vi "Autonomous Independent.vi"() -> ()   [LabVIEW 2013]
doc: "This VI is called when autonomous begins, and will automatically be terminated when autonomous ends. You can carry out timed or sensor driven robot movement independently without needing to return to the caller."
uses:
  <vilib>/addons/Kinect/Skeleton Vertex Index.ctl
  Robot Global Data.vi
  <vilib>/addons/control/pid/pid.llb/PID (DBL).vi
  <vilib>/addons/control/pid/pid.llb/PID Control Input Filter (DBL).vi
  <vilib>/addons/control/pid/NI_PID_pid.lvlib
panel:
  out "Waveform Chart 4":dbl(graph)
  out "Waveform Chart 3":dbl(graph)
  out "Waveform Chart 2":dbl(graph)
  out "Waveform Chart":dbl(graph)
  out "Autonomous \nProgram":u32
  in  "Autonomous Mode":T1(tab)
  in  "When To Fire 1":dbl=5.0
  in  "auto 3 distance":dbl=110.0
  out "test auto":i32=13
  in  "stop delay":dbl=0.5
  out "Pause":bool
  out "State 2":i32
  in  "right turn angle 2":dbl=12.0
  in  "left turn angle 2":dbl=-12.0
  in  "auto 3 distance 3":dbl=92.0
  out "Turn Left":bool
  in  "Anti Rotate":T2={"proportional gain (Kc)"=0.03, "integral time (Ti, min)"=0.01, "derivative time (Td, min)"=0.003} {"derivative time (Td, min)" format="%.3f"; "integral time (Ti, min)" format="%.3f"; "proportional gain (Kc)" format="%.3f"}
  out "Autonomous state":u32
  in  "When To Start Firing":dbl=4.95
  in  "Abort Turn":dbl=1.5
  in  "When To Start Firing 2":dbl=4.95
  in  "right turn angle 3":dbl=10.0
  in  "left turn angle 3":dbl=-20.0
  in  "auto 3 distance 5":dbl=120.0
  out "State 3":i32
  out "Turn Left 2":bool
  in  "BackupLimit":dbl=12.0
  in  "BackupSpeed":dbl=0.3 format="%#_13g"
  in  "Catapult Down":dbl=1.5 format="%#_13g"
  in  "Fire Delay":dbl format="%#_13g"
  in  "Left Rotate":dbl=-0.75
  in  "Left Strafe":dbl=-0.25 format="%#_13g"
  in  "Fire Delay 2":dbl format="%#_13g"
  in  "Catapult Down 2":dbl=1.5 format="%#_13g"
  out "State 4":i32
  in  "auto 3 distance 6":dbl=148.0
  in  "Left Strafe 2":dbl=-0.25 format="%#_13g"
  in  "Left Rotate 2":dbl=-0.75
  in  "Abort Turn 2":dbl=1.5
  out "Turn Left 3":bool
  in  "right turn angle 4":dbl=10.0
  in  "left turn angle 4":dbl=-20.0
  in  "When To Start Firing 3":dbl=4.95
  in  "BackupSpeed 2":dbl=0.3 format="%#_13g"
  in  "BackupLimit 2":dbl=36.0
  in  "Slowdown Distance":dbl=48.0
  in  "Ball Drop Distance":dbl
  in  "Catapult Down 3":dbl=1.5 format="%#_13g"
  out "State 5":i32
  in  "Ball Drop Distance 2":dbl
  in  "Slowdown Distance 2":dbl=48.0
  in  "Abort Turn 3":dbl=1.5
  out "Turn Left 4":bool
  in  "BackupSpeed 3":dbl=0.3 format="%#_13g"
  in  "BackupLimit 3":dbl=36.0
  out "State":i32
  in  "auto 3 distance 4":dbl=117.5
  in  "Track PID":T2={"proportional gain (Kc)"=0.09, "integral time (Ti, min)"=0.003, "derivative time (Td, min)"=0.001} {"derivative time (Td, min)" format="%.3f"; "integral time (Ti, min)" format="%.3f"; "proportional gain (Kc)" format="%.3f"}
  in  "Rate Thresh":dbl=500.0 step=0.001
  in  "Threshhold 2":sgl(knob)=0.75626117 scale=0.0..2.0
  out "x > y?":bool
  out "x-y 2":cluster{"x":sgl, "y":sgl, "z":sgl}
  out "Y":sgl
  # "Auto 4 Settings that work\nAuto Distance 130\nSpeed 0.75"
  # "Be sure to right-click and choose Data Operations>>Make Current Value default if you want to save the array values with the VI"
  # "PID values to use for anti rotation\nP=.03\nI=.01\nD=.003"
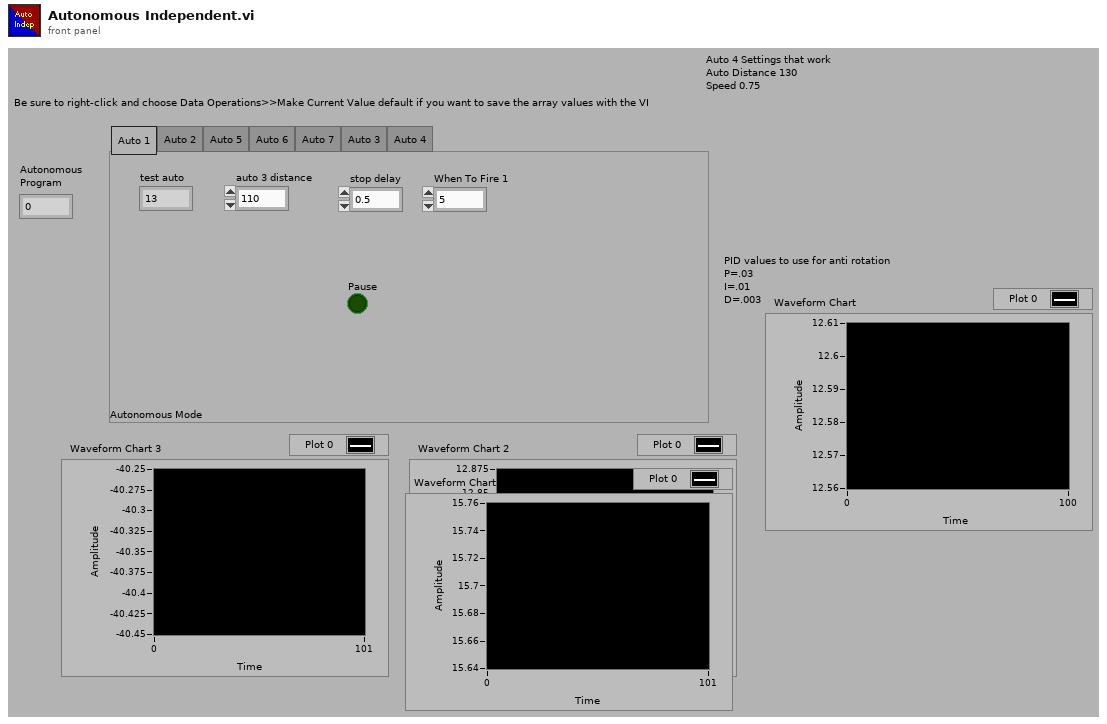
[diagram p1: front panel]
types:
  T1 = enum32{"Auto 1", "Auto 2", "Auto 5", "Auto 6", "Auto 7", "Auto 3", "Auto 4"}
  T2 = cluster{"proportional gain (Kc)":dbl, "integral time (Ti, min)":dbl, "derivative time (Td, min)":dbl}
  T3 = typedef "WPI_EncoderDevRef.ctl" = cluster{"DevStatus":errorcluster, "EncoderIndex":T4, "CounterIndex":T5, "DistancePerCount":dbl, "Decoding Type":T6}
  T4 = typedef "FPGA_EncoderIdx.ctl" = enum8{"Enc 0", "Enc 1", "Enc 2", "Enc 3", "Invalid"}
  T5 = typedef "FPGA_CounterCtrSystemIndex.ctl" = enum8{"Ctr 0", "Ctr 1", "Ctr 2", "Ctr 3", "Ctr 4", "Ctr 5", "Ctr 6", "Ctr 7", "Invalid"}
  T6 = typedef "WPI_EncoderType.ctl" = enum16{"1x", "2x", "4x"}
  T7 = typedef "WPI_GyroDevRef.ctl" = cluster{"DevStatus":errorcluster, "Analog Module":T8, "Analog Channel":T9, "Offset":dbl, "Gain (VoltsPerDegree/Second)":dbl}
  T8 = typedef "FPGA_TypedefAnalogModule.ctl" = enum16{"Analog Module 1", "Analog Module 2"}
  T9 = typedef "FPGA_AIChannel.ctl" = enum8{"AI 1", "AI 2", "AI 3", "AI 4", "AI 5", "AI 6", "AI 7", "AI 8", "Invalid"}
  T10 = typedef "WPI_AnalogChannelDevRef.ctl" = cluster{"DevStatus":errorcluster, "Analog Module":T8, "Analog Channel":T9}
  T11 = typedef "WPI_DigitalInputDevRef.ctl" = cluster{"DevStatus":errorcluster, "DIO Channel":T12, "Digital Module":T13}
  T12 = typedef "FPGA_DIOChannel.ctl" = enum8{"DIO 1", "DIO 2", "DIO 3", "DIO 4", "DIO 5", "DIO 6", "DIO 7", "DIO 8", "DIO 9", "DIO 10", "DIO 11", "DIO 12", "DIO 13", "DIO 14", "Invalid"}
  T13 = typedef "FPGA_TypedefDigitalModule.ctl" = enum16{"Digital Module 1", "Digital Module 2"}
  T14 = typedef "Skeleton Vertex Index.ctl" = i32
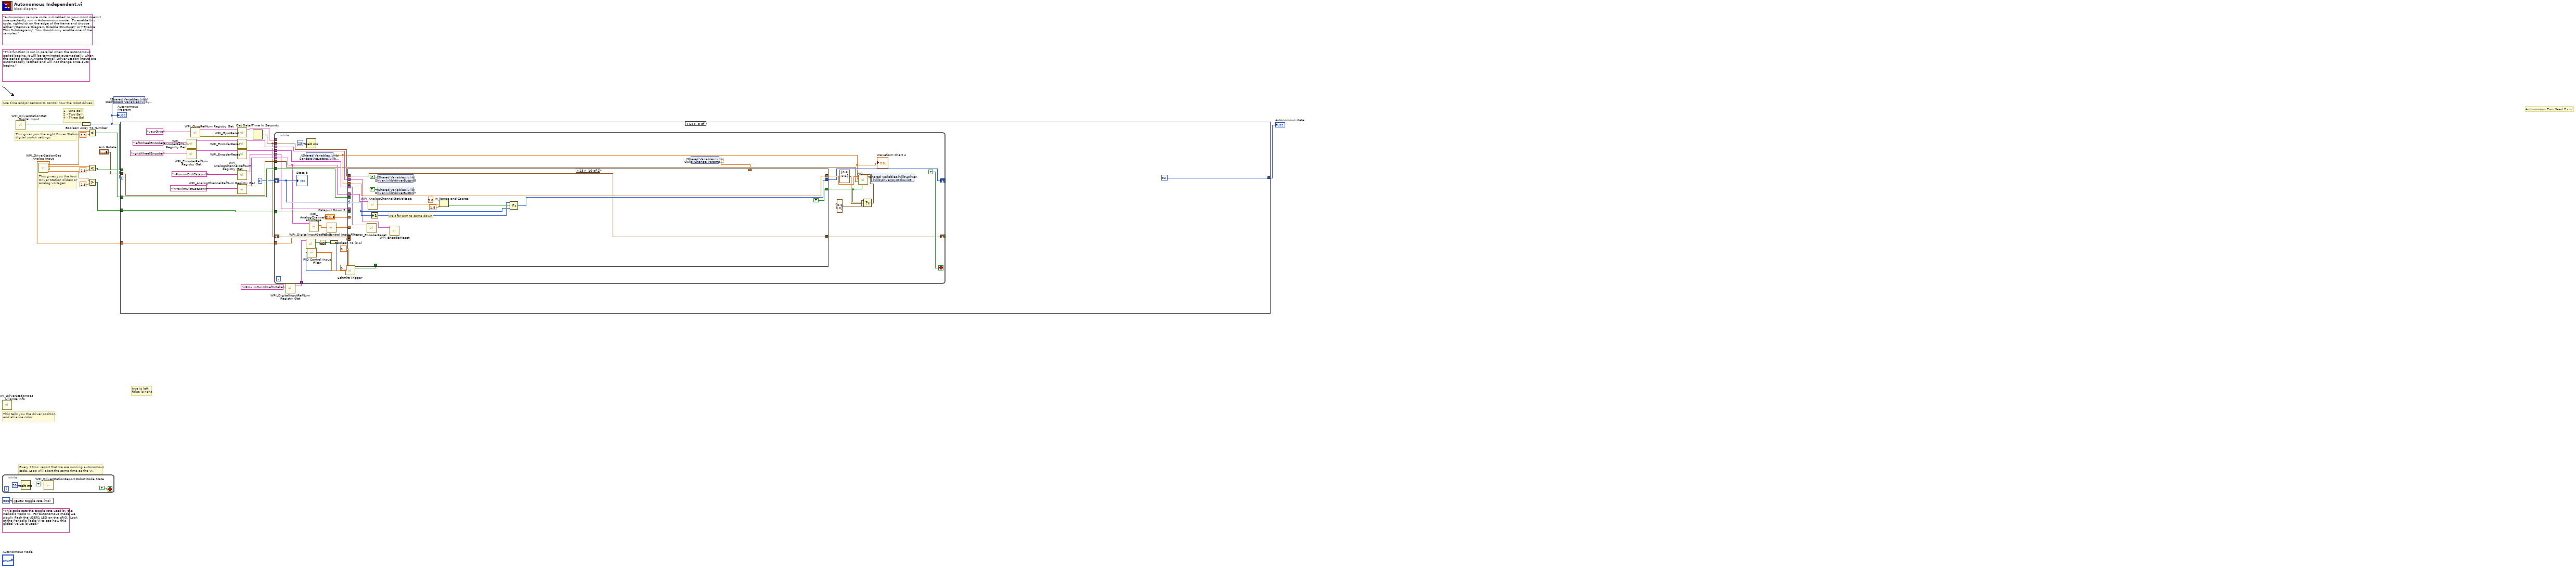
[diagram p0: block diagram]
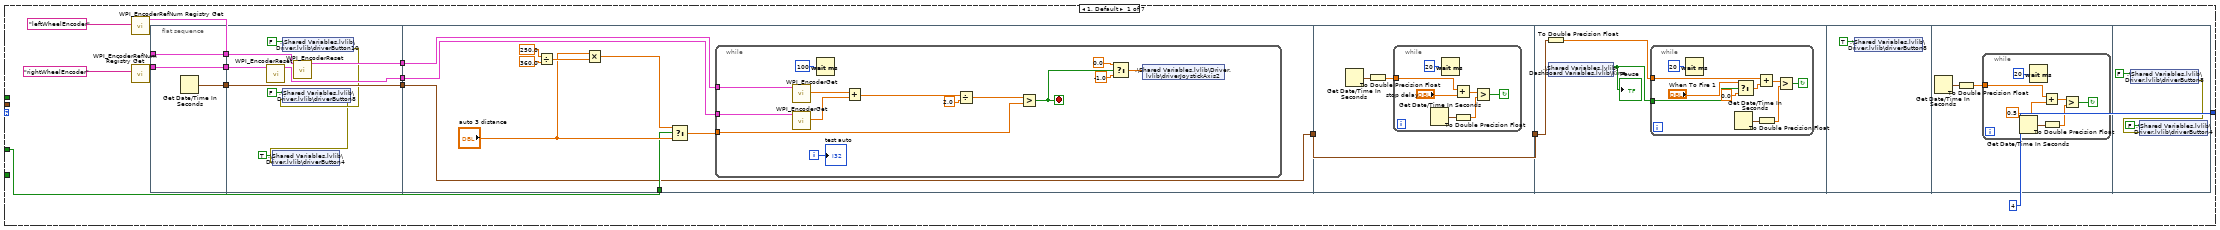
[diagram p2: hidden frame]
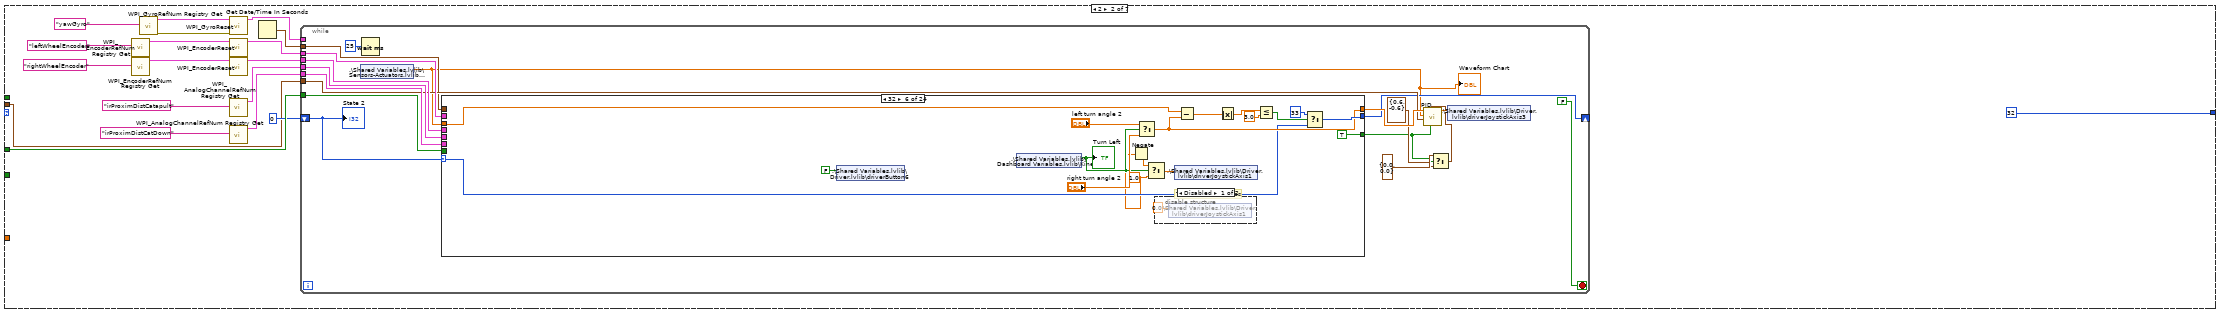
[diagram p3: hidden frame]
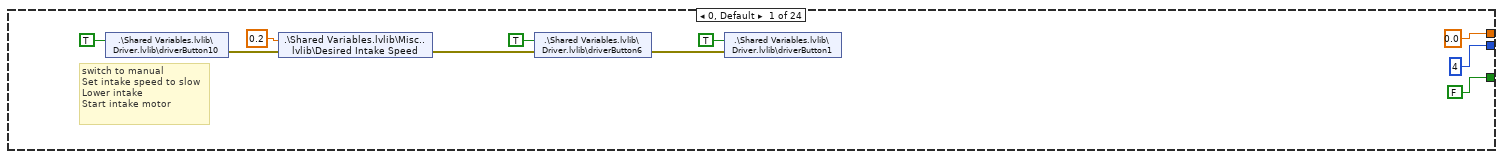
[diagram p4: hidden frame]
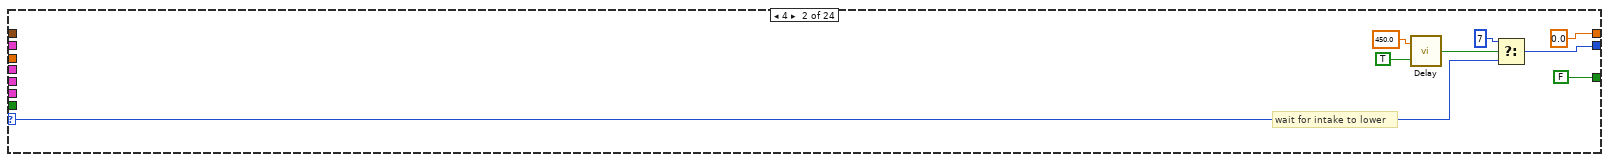
[diagram p5: hidden frame]
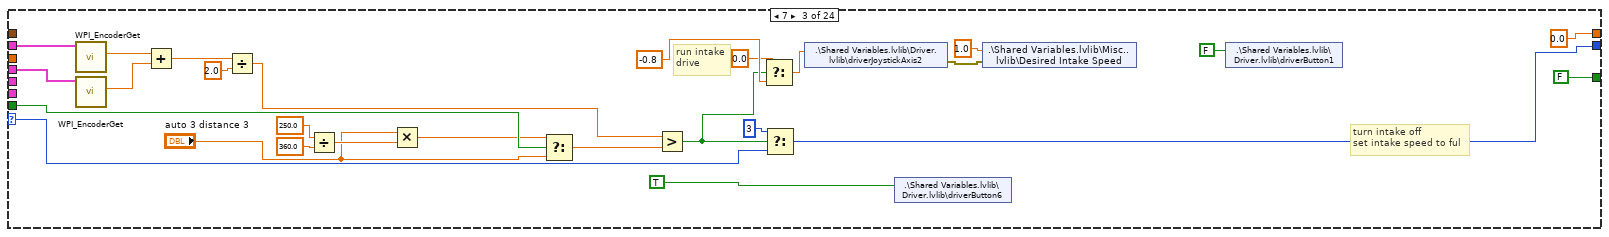
[diagram p6: hidden frame]
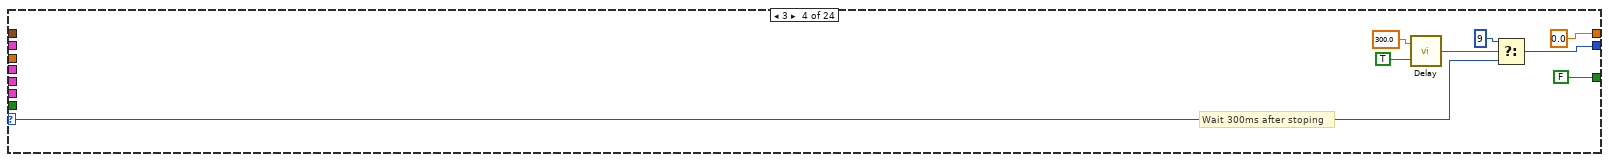
[diagram p7: hidden frame]
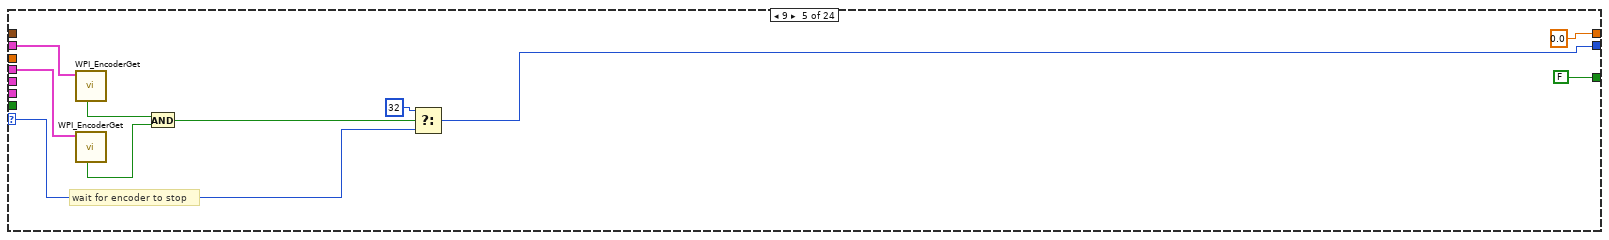
[diagram p8: hidden frame]
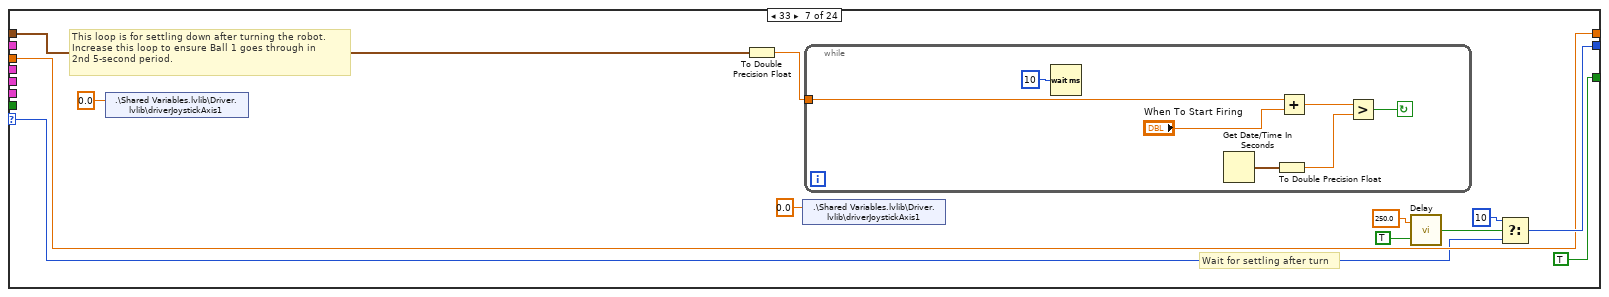
[diagram p10: hidden frame]
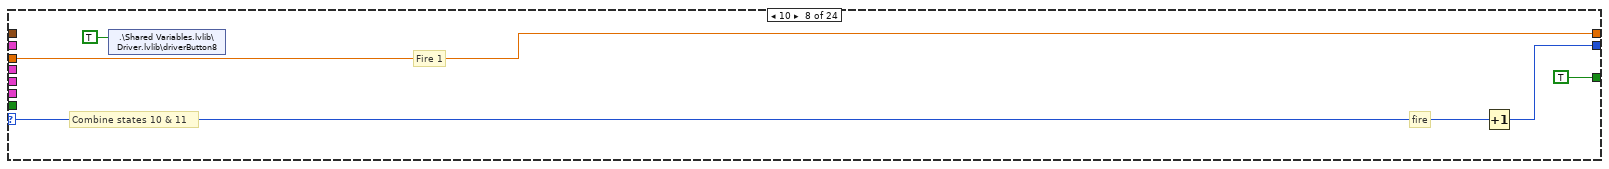
[diagram p11: hidden frame]
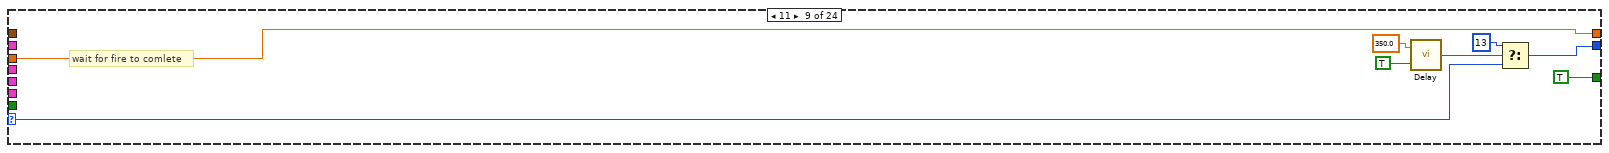
[diagram p12: hidden frame]
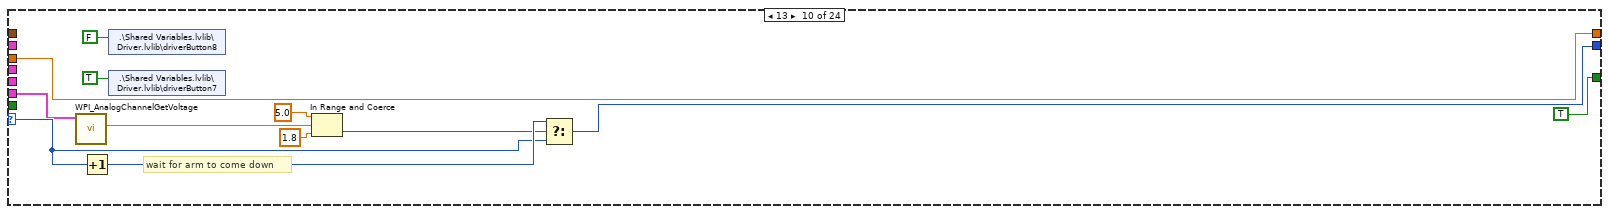
[diagram p13: hidden frame]
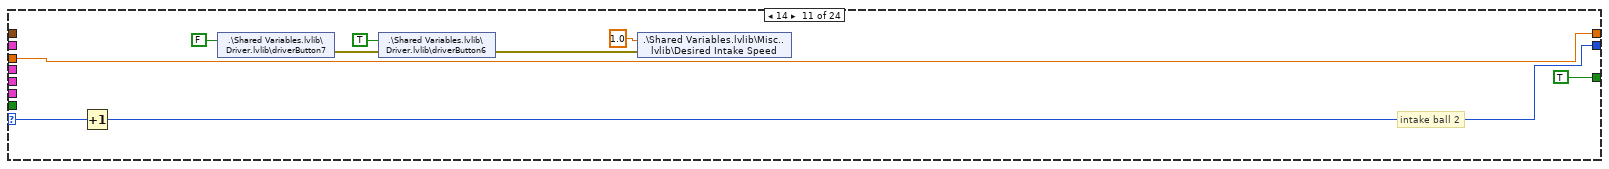
[diagram p14: hidden frame]
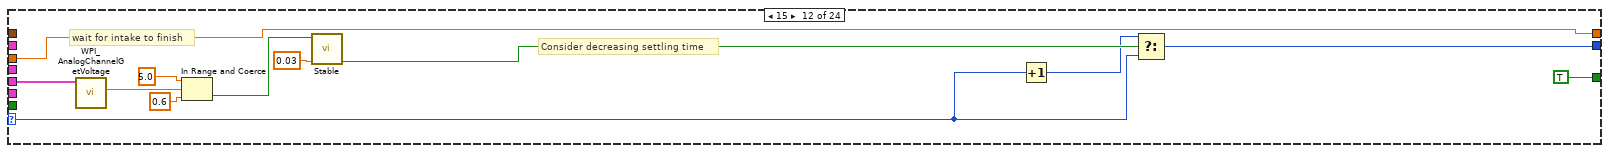
[diagram p15: hidden frame]
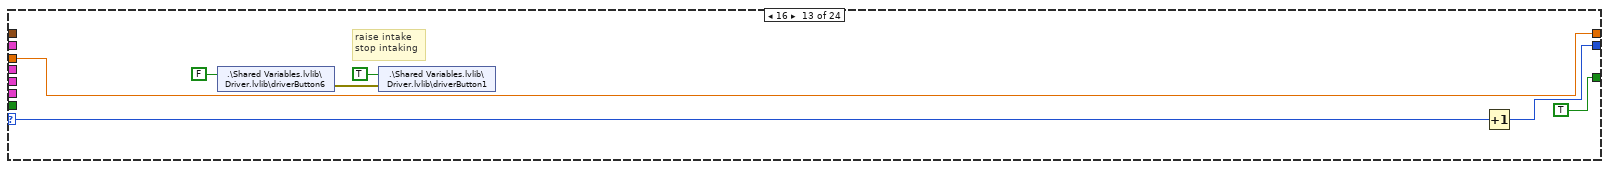
[diagram p16: hidden frame]
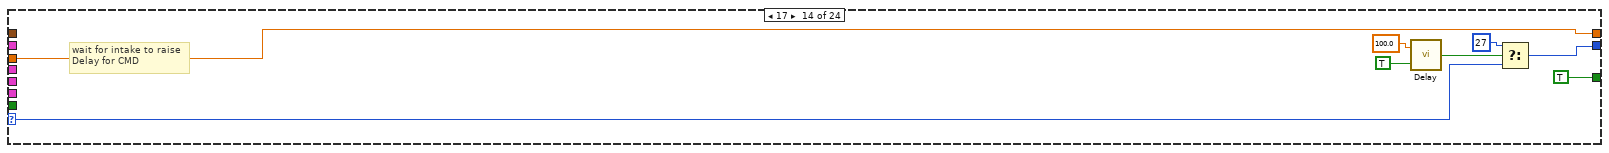
[diagram p17: hidden frame]
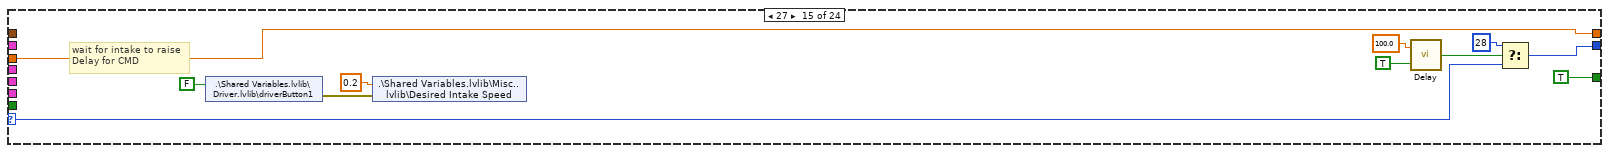
[diagram p18: hidden frame]
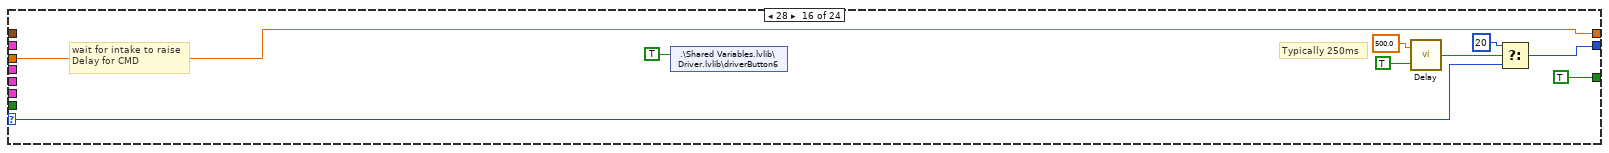
[diagram p19: hidden frame]
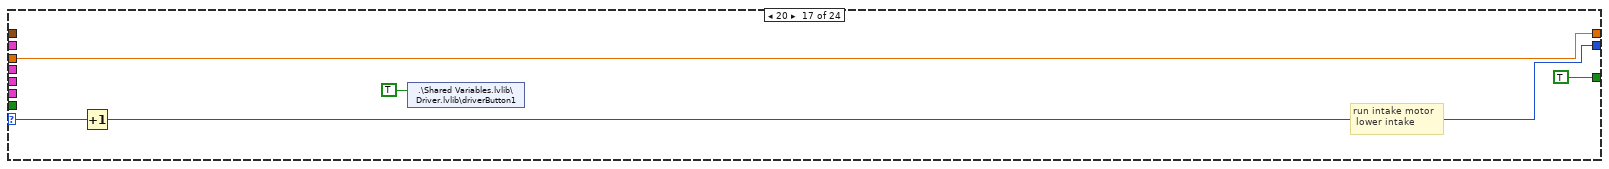
[diagram p20: hidden frame]
diagram:
  (unwired) "This code sets the toggle rate used by the Periodic Tasks VI.  For autonomous mode we slowly flash the USER1 LED on the cRIO.  Look at the Periodic Tasks VI to see how this global value is used."
  (unwired) "Autonomous sample code is disabled so your robot doesn't unexpectantly run in Autonomous mode.  To enable this code, right-click on the edge of the frame and choose either \"Remove Diagram Disable Structure\" or \"Enable This Subdiagram\". You should only enable one of the samples."
  (unwired) "This function is run in parallel when the autonomous period begins. It will be terminated automatically when the period ends.\n\nNote that all Driver Station inputs are automatically latched and will not change once auto begins."
  # "1 - One Ball\n2 - Two Ball\n4 - Three Bal"
  # "true is left\nfalse is right"
  # "Autonomous Two Need Fixin'"
  # "This gives you the eight Driver Station\ndigital switch settings"
  # "Every 20ms, report that we are running autonomous\ncode. Loop will abort the same time as the VI."
  # "Use time and/or sensors to control how the robot drives."
  # "This tells you the driver position\nand alliance color"
  # "This gives you the four\nDriver Station sliders or\nanalog voltages"
  n1 = call <vilib>:"WPI_DriverStationGet Alliance Info.vi"() -> ()  [unwired: 12 out]
  n2 = while {
    stop <- FALSE stop-if-true
    n3 = Wait (ms)(milliseconds to wait=u32 20) -> ()  [unwired: 1 out]
    n4 = call <vilib>:"WPI_DriverStationReport Robot Code State.vi"("Autonomous"=TRUE) -> ()  [unwired: 10 in, 1 out]
  }
  n5 = global write "Robot Global Data.vi" "LED toggle rate (ms)"(u32 500 ("LED ms toggle rate")) -> ()
  n6 = call <vilib>:"WPI_DriverStationGet Digital Input.vi"() -> ("Driver Station Digital Input (1-8)"=w14:bool[])  [unwired: 11 out]
  n7 = call <vilib>:"WPI_DriverStationGet Analog Input.vi"() -> ("Analog 4 (V)"=w3:dbl, "Analog 3 (V)"=w1:dbl, "Analog 2 (V)"=w7:dbl, "Analog 1 (V)"=w12:dbl)  [unwired: 8 out]
  n8 = Boolean Array To Number(Boolean array=w14) -> (number=w5:u32)
  "Autonomous \nProgram" <- w5
  n9 = Less?(x=w12, y=2.5) -> (x < y?=w10:bool)
  n10 = Less?(x=w7, y=2.5) -> (x < y?=w8:bool)
  n11 = Greater?(x=w3, y=2.5) -> (0:w2:bool)
  n12 = shared-variable ".\\Shared Variables.lvlib\\Dashboard Variables.lvlib\\Auto Mode"(w5) -> ()  [unwired: 1 in, 1 out]
  n13 = case shown="64" w5 {
    selector: w5 -> [_ _ _ _ _ _ w1912]
    tunnel: [4 32 32 32 32 16 w1912] -> w13
    tunnel: w10 -> [w25 w119 w398 w759 w1163 w1553 _]
    tunnel: w8 -> [_ _ _ _ _ w1564 _]
    tunnel: "Anti Rotate" -> [_ w107 w386 w747 w1151 w1559 _]
    tunnel: w2 -> [_ _ w382 w743 w1147 _ _]
    tunnel: w1 -> [_ _ w381 w742 w1146 _ _]
    frame 1, Default {
      n14 = call <vilib>:"WPI_EncoderRefNum Registry Get.vi"("refnum name"="leftWheelEncoder") -> ("EncoderDevRef"=w31:T3)  [unwired: 9 in, 1 out]
      n15 = call <vilib>:"WPI_EncoderRefNum Registry Get.vi"("refnum name"="rightWheelEncoder") -> ("EncoderDevRef"=w30:T3)  [unwired: 9 in, 1 out]
      n16 = flat-sequence {
        tunnel: w30 -> [w34]
        tunnel: w31 -> [w35]
        tunnel: [w35] -> w24
        tunnel: [w34] -> w23
        tunnel: [w33] -> w19
        tunnel: [w43] -> w27
        tunnel: [w42] -> w26
        tunnel: w24 -> [w45]
        tunnel: w23 -> [w44]
        tunnel: [w39] -> w20
        tunnel: w19 -> [w39]
        tunnel: w27 -> [w55]
        tunnel: w26 -> [w54]
        tunnel: w25 -> [w49]
        tunnel: [w46] -> w21
        tunnel: w20 -> [w46]
        tunnel: [w70] -> w22
        tunnel: w21 -> [w70]
        tunnel: w22 -> [w80]
        frame #0 {
          n17 = Get Date/Time In Seconds() -> (seconds since 1Jan1904=w33:timestamp)
        }
        frame #1 {
          n18 = call <vilib>:"WPI_EncoderReset.vi"("EncoderDevRef"=w44) -> ("EncoderDevRef"=w43:T3)  [unwired: 9 in, 1 out]
          n19 = shared-variable ".\\Shared Variables.lvlib\\Driver.lvlib\\driverButton10"(FALSE ("driverButton10")) -> (error out=w38:errorcluster)  [unwired: 1 in]
          n20 = shared-variable ".\\Shared Variables.lvlib\\Driver.lvlib\\driverButton8"(FALSE ("driverButton1"), error in=w38) -> (error out=w37:errorcluster)
          n21 = shared-variable ".\\Shared Variables.lvlib\\Driver.lvlib\\driverButton4"(TRUE ("driverButton4"), error in=w37) -> ()  [unwired: 1 out]
          n22 = call <vilib>:"WPI_EncoderReset.vi"("EncoderDevRef"=w45) -> ("EncoderDevRef"=w42:T3)  [unwired: 9 in, 1 out]
        }
        frame #2 {
          n23 = Divide(x=250.0, y=360.0) -> (x/y=w51:dbl)
          n24 = Multiply(x="auto 3 distance", y=w51) -> (x*y=w53:dbl)
          n25 = Select(t=w53, s=w49, f="auto 3 distance") -> (s? t:f=w48:dbl)
          n26 = while {
            tunnel: w55 -> [w63]
            tunnel: w54 -> [w62]
            tunnel: w48 -> [w56]
            i -> [w64]
            stop <- w66 stop-if-true
            n27 = call <vilib>:"WPI_EncoderGet.vi"("EncoderDevRef"=w62) -> ("Distance"=w61:dbl)  [unwired: 5 in, 5 out]
            n28 = call <vilib>:"WPI_EncoderGet.vi"("EncoderDevRef"=w63) -> ("Distance"=w60:dbl)  [unwired: 5 in, 5 out]
            n29 = Wait (ms)(milliseconds to wait=u32 100) -> ()  [unwired: 1 out]
            n30 = Add(x=w61, y=w60) -> (x+y=w59:dbl)
            n31 = Divide(x=w59, y=2.0) -> (x/y=w57:dbl)
            n32 = Greater?(x=w57, y=w56) -> (0:w66:bool)
            n33 = Select(t=0.0, s=w66, f=-1.0) -> (s? t:f=w67:dbl)
            n34 = shared-variable ".\\Shared Variables.lvlib\\Driver.lvlib\\driverJoystickAxis2"(w67) -> ()  [unwired: 1 in, 1 out]
            "test auto" <- w64
          }
        }
        frame #3 {
          n35 = Get Date/Time In Seconds() -> (seconds since 1Jan1904=w72:timestamp)
          n36 = To Double Precision Float(number=w72) -> (double precision float=w71:dbl)
          n37 = while {
            tunnel: w71 -> [w73]
            stop <- w76 continue-if-true
            n38 = Get Date/Time In Seconds() -> (seconds since 1Jan1904=w79:timestamp)
            n39 = Wait (ms)(milliseconds to wait=u32 20) -> ()  [unwired: 1 out]
            n40 = Add(x=w73, y="stop delay") -> (x+y=w78:dbl)
            n41 = To Double Precision Float(number=w79) -> (double precision float=w77:dbl)
            n42 = Greater?(x=w78, y=w77) -> (0:w76:bool)
          }
        }
        frame #4 {
          n43 = To Double Precision Float(number=w80) -> (double precision float=w82:dbl)
          n44 = shared-variable ".\\Shared Variables.lvlib\\Dashboard Variables.lvlib\\Kinect Status"() -> (w81:bool)  [unwired: 1 in, 1 out]
          "Pause" <- w81
          n45 = while {
            tunnel: w82 -> [w92]
            tunnel: w81 -> [w87]
            stop <- w88 continue-if-true
            n46 = Wait (ms)(milliseconds to wait=u32 20) -> ()  [unwired: 1 out]
            n47 = Get Date/Time In Seconds() -> (seconds since 1Jan1904=w91:timestamp)
            n48 = Select(t="When To Fire 1", s=w87, f=0.0) -> (s? t:f=w86:dbl)
            n49 = Add(x=w92, y=w86) -> (x+y=w90:dbl)
            n50 = To Double Precision Float(number=w91) -> (double precision float=w89:dbl)
            n51 = Greater?(x=w90, y=w89) -> (0:w88:bool)
          }
        }
        frame #5 {
          n52 = shared-variable ".\\Shared Variables.lvlib\\Driver.lvlib\\driverButton8"(TRUE ("driverButton1")) -> ()  [unwired: 1 in, 1 out]
        }
        frame #6 {
          n53 = Get Date/Time In Seconds() -> (seconds since 1Jan1904=w94:timestamp)
          n54 = To Double Precision Float(number=w94) -> (double precision float=w95:dbl)
          n55 = while {
            tunnel: w95 -> [w96]
            stop <- w99 continue-if-true
            n56 = Get Date/Time In Seconds() -> (seconds since 1Jan1904=w102:timestamp)
            n57 = Wait (ms)(milliseconds to wait=u32 20) -> ()  [unwired: 1 out]
            n58 = Add(x=w96, y=0.5 ("stop delay 2")) -> (x+y=w101:dbl)
            n59 = To Double Precision Float(number=w102) -> (double precision float=w100:dbl)
            n60 = Greater?(x=w101, y=w100) -> (0:w99:bool)
          }
        }
        frame #7 {
          n61 = shared-variable ".\\Shared Variables.lvlib\\Driver.lvlib\\driverButton8"(FALSE ("driverButton1")) -> (error out=w103:errorcluster)  [unwired: 1 in]
          n62 = shared-variable ".\\Shared Variables.lvlib\\Driver.lvlib\\driverButton4"(FALSE ("driverButton4"), error in=w103) -> ()  [unwired: 1 out]
        }
      }
    }
    frame 2 {
      n63 = call <vilib>:"WPI_EncoderRefNum Registry Get.vi"("refnum name"="leftWheelEncoder") -> ("EncoderDevRef"=w123:T3)  [unwired: 9 in, 1 out]
      n64 = call <vilib>:"WPI_EncoderRefNum Registry Get.vi"("refnum name"="rightWheelEncoder") -> ("EncoderDevRef"=w122:T3)  [unwired: 9 in, 1 out]
      n65 = call <vilib>:"WPI_GyroRefNum Registry Get.vi"("refnum name"="yawGyro") -> ("error out"=w110:errorcluster, "GyroDevRef"=w111:T7)  [unwired: 9 in]
      n66 = call <vilib>:"WPI_GyroReset.vi"("error in (no error)"=w110, "GyroDevRef"=w111) -> ("GyroDevRef"=w108:T7)  [unwired: 8 in, 1 out]
      n67 = call <vilib>:"WPI_EncoderReset.vi"("EncoderDevRef"=w123) -> ("EncoderDevRef"=w118:T3)  [unwired: 9 in, 1 out]
      n68 = call <vilib>:"WPI_EncoderReset.vi"("EncoderDevRef"=w122) -> ("EncoderDevRef"=w117:T3)  [unwired: 9 in, 1 out]
      n69 = call <vilib>:"WPI_AnalogChannelRefNum Registry Get.vi"("refnum name"="irProximDistCatapult") -> ("AIDeviceRef"=w116:T10)  [unwired: 9 in, 1 out]
      n70 = call <vilib>:"WPI_AnalogChannelRefNum Registry Get.vi"("refnum name"="irProximDistCatDown") -> ("AIDeviceRef"=w112:T10)  [unwired: 9 in, 1 out]
      n71 = Get Date/Time In Seconds() -> (seconds since 1Jan1904=w106:timestamp)
      n72 = while {
        tunnel: w119 -> [w142]
        tunnel: w118 -> [w141]
        tunnel: w117 -> [w140]
        tunnel: w116 -> [w137]
        shift-right: [w132] -> _
        shift-left: 0 -> [w136]
        tunnel: w112 -> [w135]
        tunnel: w108 -> [_]
        tunnel: w107 -> [w133]
        tunnel: w106 -> [w130]
        stop <- FALSE stop-if-true
        n73 = shared-variable ".\\Shared Variables.lvlib\\Sensors-Actuators.lvlib\\Gyro.lvlib\\yawGyro"() -> (w125:dbl)  [unwired: 1 in, 1 out]
        "Waveform Chart" <- w125
        n74 = Wait (ms)(milliseconds to wait=u32 25) -> ()  [unwired: 1 out]
        n75 = case shown="32" w136 {
          selector: w136 -> [_ w156 w172 w192 w205 w213 w231 w246 w252 w266 w275 w281 w294 w300 w311 w320 w328 w332 w342 w349 w358 w368 w371 w379]
          tunnel: [4 ("t") w158 w184 w191 w204 w220 w234 w245 w251 w265 w274 w279 w293 w299 w310 w319 w327 w331 w341 w348 w357 w369 w371 w379] -> w132
          tunnel: w142 -> [_ _ w187 _ _ _ _ _ _ _ _ _ _ _ _ _ _ _ _ _ _ _ _ _]
          tunnel: w141 -> [_ _ w186 _ w203 _ _ _ _ _ _ _ _ _ _ _ _ _ _ _ _ _ _ _]
          tunnel: w140 -> [_ _ w185 _ w202 _ _ _ _ _ _ _ _ _ _ _ _ _ _ _ _ _ _ _]
          tunnel: w137 -> [_ _ _ _ _ _ _ _ _ _ _ w288 _ _ _ _ _ _ _ _ _ _ _ _]
          tunnel: w135 -> [_ _ _ _ _ _ _ _ _ w264 _ _ _ _ _ _ _ _ _ _ _ w363 _ _]
          tunnel: [0.0 ("setpoint") 0.0 ("setpoint") 0.0 ("setpoint") 0.0 ("setpoint") 0.0 ("setpoint") w218 w233 w244 w250 w259 w271 w278 w290 w298 w309 w318 w326 w330 w338 w347 w355 w362 w373 w378] -> w134
          tunnel: w125 -> [_ _ _ _ _ w219 w233 w244 w250 w259 w271 w278 w290 w298 w309 w318 w326 w330 w338 w347 w355 w362 w373 w378]
          tunnel: [FALSE FALSE FALSE FALSE FALSE TRUE TRUE TRUE TRUE TRUE TRUE TRUE TRUE TRUE TRUE TRUE TRUE TRUE TRUE TRUE TRUE TRUE TRUE FALSE] -> w126
          tunnel: w130 -> [_ _ _ _ _ _ w225 _ _ _ _ _ _ _ _ _ _ _ _ _ _ _ _ _]
          frame 0, Default {
            # "switch to manual\nSet intake speed to slow\nLower intake\nStart intake motor"
            n76 = shared-variable ".\\Shared Variables.lvlib\\Driver.lvlib\\driverButton10"(TRUE ("driverButton10")) -> (error out=w144:errorcluster)  [unwired: 1 in]
            n77 = shared-variable ".\\Shared Variables.lvlib\\Misc..lvlib\\Desired Intake Speed"(0.2 ("Intake RPM"), error in=w144) -> (error out=w143:errorcluster)
            n78 = shared-variable ".\\Shared Variables.lvlib\\Driver.lvlib\\driverButton6"(TRUE ("driverButton6"), error in=w143) -> (error out=w146:errorcluster)
            n79 = shared-variable ".\\Shared Variables.lvlib\\Driver.lvlib\\driverButton1"(TRUE ("driverButton1"), error in=w146) -> ()  [unwired: 1 out]
          }
          frame 4 {
            # "wait for intake to lower"
            n80 = call "Delay.vi"("Timer Going?"=TRUE, "Time to Wait (ms)"=450.0) -> ("Time Up"=w159:bool)
            n81 = Select(t=7, s=w159, f=w156) -> (s? t:f=w158:i32)
          }
          frame 7 {
            # "turn intake off\nset intake speed to ful"
            # "run intake\ndrive"
            n82 = call <vilib>:"WPI_EncoderGet.vi"("EncoderDevRef"=w186) -> ("Distance"=w178:dbl)  [unwired: 5 in, 5 out]
            n83 = call <vilib>:"WPI_EncoderGet.vi"("EncoderDevRef"=w185) -> ("Distance"=w177:dbl)  [unwired: 5 in, 5 out]
            n84 = Add(x=w178, y=w177) -> (x+y=w176:dbl)
            n85 = Divide(x=w176, y=2.0) -> (x/y=w174:dbl)
            n86 = Divide(x=250.0, y=360.0) -> (x/y=w181:dbl)
            n87 = Multiply(x="auto 3 distance 3", y=w181) -> (x*y=w183:dbl)
            n88 = Select(t=w183, s=w187, f="auto 3 distance 3") -> (s? t:f=w173:dbl)
            n89 = Greater?(x=w174, y=w173) -> (0:w162:bool)
            n90 = Select(t=0.0, s=w162, f=-0.8 ("driverJoystickAxis2")) -> (s? t:f=w163:dbl)
            n91 = Select(t=3, s=w162, f=w172) -> (s? t:f=w184:i32)
            n92 = shared-variable ".\\Shared Variables.lvlib\\Driver.lvlib\\driverJoystickAxis2"(w163) -> (error out=w161:errorcluster)  [unwired: 1 in]
            n93 = shared-variable ".\\Shared Variables.lvlib\\Driver.lvlib\\driverButton6"(TRUE ("driverButton6")) -> ()  [unwired: 1 in, 1 out]
            n94 = shared-variable ".\\Shared Variables.lvlib\\Misc..lvlib\\Desired Intake Speed"(1.0 ("Desired Intake Speed"), error in=w161) -> ()  [unwired: 1 out]
            n95 = shared-variable ".\\Shared Variables.lvlib\\Driver.lvlib\\driverButton1"(FALSE ("driverButton1")) -> ()  [unwired: 1 in, 1 out]
          }
          frame 3 {
            # "Wait 300ms after stoping"
            n96 = call "Delay.vi"("Timer Going?"=TRUE, "Time to Wait (ms)"=300.0) -> ("Time Up"=w194:bool)
            n97 = Select(t=9 ("x"), s=w194, f=w192) -> (s? t:f=w191:i32)
          }
          frame 9 {
            # "wait for encoder to stop"
            n98 = call <vilib>:"WPI_EncoderGet.vi"("EncoderDevRef"=w203) -> ("Stopped"=w201:bool)  [unwired: 5 in, 5 out]
            n99 = call <vilib>:"WPI_EncoderGet.vi"("EncoderDevRef"=w202) -> ("Stopped"=w200:bool)  [unwired: 5 in, 5 out]
            n100 = And(x=w201, y=w200) -> (x .and. y?=w199:bool)
            n101 = Select(t=32, s=w199, f=w205) -> (s? t:f=w204:i32)
          }
          frame 32 {
            w207 = 1.0 ("f")
            # "Turn robot X degrees"
            n102 = shared-variable ".\\Shared Variables.lvlib\\Driver.lvlib\\driverButton6"(FALSE ("driverButton6")) -> ()  [unwired: 1 in, 1 out]
            n103 = shared-variable ".\\Shared Variables.lvlib\\Dashboard Variables.lvlib\\Kinect Status"() -> (w209:bool)  [unwired: 1 in, 1 out]
            "Turn Left" <- w209
            n104 = Negate(x=w207) -> (-x=w208:dbl)
            n105 = Select(t="left turn angle 2", s=w209, f="right turn angle 2") -> (s? t:f=w218:dbl)
            n106 = Select(t=w208, s=w209, f=w207) -> (s? t:f=w210:dbl)
            n107 = disable-structure shown="Disabled" {
              frame Disabled {
                n108 = shared-variable ".\\Shared Variables.lvlib\\Driver.lvlib\\driverJoystickAxis1"(0.0 ("driverJoystickAxis1")) -> ()  [unwired: 1 in, 1 out]
              }
              frame Enabled {
              }
            }
            n109 = shared-variable ".\\Shared Variables.lvlib\\Driver.lvlib\\driverJoystickAxis1"(w210) -> ()  [unwired: 1 in, 1 out]
            n110 = Subtract(x=w219, y=w218) -> (x-y=w217:dbl)
            n111 = Absolute Value(x=w217) -> (abs(x)=w216:dbl)
            n112 = Less Or Equal?(x=w216, y=3.0) -> (x <= y?=w214:bool)
            n113 = Select(t=33, s=w214, f=w213) -> (s? t:f=w220:i32)
          }
          frame 33 {
            # "This loop is for settling down after turning the robot.\nIncrease this loop to ensure Ball 1 goes through in \n2nd 5-second period."
            # "Wait for settling after turn"
            n114 = shared-variable ".\\Shared Variables.lvlib\\Driver.lvlib\\driverJoystickAxis1"(0.0 ("driverJoystickAxis1")) -> ()  [unwired: 1 in, 1 out]
            n115 = To Double Precision Float(number=w225) -> (double precision float=w226:dbl)
            n116 = shared-variable ".\\Shared Variables.lvlib\\Driver.lvlib\\driverJoystickAxis1"(0.0 ("driverJoystickAxis1")) -> ()  [unwired: 1 in, 1 out]
            n117 = while {
              tunnel: w226 -> [w236]
              stop <- w239 continue-if-true
              n118 = Wait (ms)(milliseconds to wait=u32 10) -> ()  [unwired: 1 out]
              n119 = Get Date/Time In Seconds() -> (seconds since 1Jan1904=w242:timestamp)
              n120 = To Double Precision Float(number=w242) -> (double precision float=w240:dbl)
              n121 = Add(x=w236, y="When To Start Firing") -> (x+y=w241:dbl)
              n122 = Greater?(x=w241, y=w240) -> (0:w239:bool)
            }
            n123 = call "Delay.vi"("Timer Going?"=TRUE, "Time to Wait (ms)"=250.0) -> ("Time Up"=w228:bool)
            n124 = Select(t=10, s=w228, f=w231) -> (s? t:f=w234:i32)
          }
          frame 10 {
            # "Combine states 10 & 11"
            # "Fire 1"
            # "fire"
            n125 = shared-variable ".\\Shared Variables.lvlib\\Driver.lvlib\\driverButton8"(TRUE ("driverButton8")) -> ()  [unwired: 1 in, 1 out]
            n126 = Increment(x=w246) -> (x+1=w245:i32)
          }
          frame 11 {
            # "wait for fire to comlete"
            n127 = call "Delay.vi"("Timer Going?"=TRUE, "Time to Wait (ms)"=350.0) -> ("Time Up"=w254:bool)
            n128 = Select(t=13, s=w254, f=w252) -> (s? t:f=w251:i32)
          }
          frame 13 {
            # "wait for arm to come down"
            n129 = call <vilib>:"WPI_AnalogChannelGetVoltage.vi"("AIDeviceRef"=w264) -> ("Voltage"=w263:dbl)  [unwired: 8 in, 2 out]
            n130 = Increment(x=w266) -> (x+1=w267:i32)
            n131 = shared-variable ".\\Shared Variables.lvlib\\Driver.lvlib\\driverButton8"(FALSE ("driverButton8")) -> ()  [unwired: 1 in, 1 out]
            n132 = shared-variable ".\\Shared Variables.lvlib\\Driver.lvlib\\driverButton7"(TRUE ("driverButton8")) -> ()  [unwired: 1 in, 1 out]
            n133 = In Range and Coerce(upper limit=5.0, x=w263, lower limit=1.8) -> (In Range?=w260:bool)  [unwired: 1 out]
            n134 = Select(t=w267, s=w260, f=w266) -> (s? t:f=w265:i32)
          }
          frame 14 {
            # "intake ball 2"
            n135 = Increment(x=w275) -> (x+1=w274:i32)
            n136 = shared-variable ".\\Shared Variables.lvlib\\Driver.lvlib\\driverButton7"(FALSE ("driverButton8")) -> (error out=w272:errorcluster)  [unwired: 1 in]
            n137 = shared-variable ".\\Shared Variables.lvlib\\Driver.lvlib\\driverButton6"(TRUE ("driverButton1"), error in=w272) -> (error out=w268:errorcluster)
            n138 = shared-variable ".\\Shared Variables.lvlib\\Misc..lvlib\\Desired Intake Speed"(1.0 ("Desired Intake Speed"), error in=w268) -> ()  [unwired: 1 out]
          }
          frame 15 {
            # "Consider decreasing settling time"
            # "wait for intake to finish"
            n139 = call <vilib>:"WPI_AnalogChannelGetVoltage.vi"("AIDeviceRef"=w288) -> ("Voltage"=w287:dbl)  [unwired: 8 in, 2 out]
            n140 = In Range and Coerce(upper limit=5.0, x=w287, lower limit=0.6) -> (In Range?=w284:bool)  [unwired: 1 out]
            n141 = call "Stable.vi"("Eval Period (sec)"=0.03, "Signal Input"=w284) -> ("Stable"=w282:bool)  [unwired: 9 in]
            n142 = Increment(x=w281) -> (x+1=w280:i32)
            n143 = Select(t=w280, s=w282, f=w281) -> (s? t:f=w279:i32)
          }
          frame 16 {
            # "raise intake\nstop intaking"
            n144 = shared-variable ".\\Shared Variables.lvlib\\Driver.lvlib\\driverButton6"(FALSE ("driverButton1")) -> (error out=w291:errorcluster)  [unwired: 1 in]
            n145 = shared-variable ".\\Shared Variables.lvlib\\Driver.lvlib\\driverButton1"(TRUE ("driverButton1"), error in=w291) -> ()  [unwired: 1 out]
            n146 = Increment(x=w294) -> (x+1=w293:i32)
          }
          frame 17 {
            # "wait for intake to raise\nDelay for CMD"
            n147 = call "Delay.vi"("Timer Going?"=TRUE, "Time to Wait (ms)"=100.0) -> ("Time Up"=w302:bool)
            n148 = Select(t=27, s=w302, f=w300) -> (s? t:f=w299:i32)
          }
          frame 27 {
            # "wait for intake to raise\nDelay for CMD"
            n149 = shared-variable ".\\Shared Variables.lvlib\\Driver.lvlib\\driverButton1"(FALSE ("driverButton1")) -> (error out=w304:errorcluster)  [unwired: 1 in]
            n150 = shared-variable ".\\Shared Variables.lvlib\\Misc..lvlib\\Desired Intake Speed"(0.2 ("Desired Intake Speed"), error in=w304) -> ()  [unwired: 1 out]
            n151 = call "Delay.vi"("Timer Going?"=TRUE, "Time to Wait (ms)"=100.0) -> ("Time Up"=w313:bool)
            n152 = Select(t=28, s=w313, f=w311) -> (s? t:f=w310:i32)
          }
          frame 28 {
            # "Typically 250ms"
            # "wait for intake to raise\nDelay for CMD"
            n153 = shared-variable ".\\Shared Variables.lvlib\\Driver.lvlib\\driverButton6"(TRUE ("driverButton1")) -> ()  [unwired: 1 in, 1 out]
            n154 = call "Delay.vi"("Timer Going?"=TRUE, "Time to Wait (ms)"=500.0) -> ("Time Up"=w322:bool)
            n155 = Select(t=20, s=w322, f=w320) -> (s? t:f=w319:i32)
          }
          frame 20 {
            # "run intake motor\n lower intake"
            n156 = Increment(x=w328) -> (x+1=w327:i32)
            n157 = shared-variable ".\\Shared Variables.lvlib\\Driver.lvlib\\driverButton1"(TRUE ("driverButton1")) -> ()  [unwired: 1 in, 1 out]
          }
          frame 21 {
            # "Consider decreasing settling time"
            # "wait for intake to lower\n(450ms)"
            n158 = Increment(x=w332) -> (x+1=w335:i32)
            n159 = call "Delay.vi"("Timer Going?"=TRUE, "Time to Wait (ms)"=450.0 ("Wait for Intake to Lower (450ms)")) -> ("Time Up"=w334:bool)
            n160 = Select(t=w335, s=w334, f=w332) -> (s? t:f=w331:i32)
          }
          frame 22 {
            # "stop running intake motor\nfire\nDe-Assert Lower Intake"
            n161 = Increment(x=w342) -> (x+1=w341:i32)
            n162 = shared-variable ".\\Shared Variables.lvlib\\Driver.lvlib\\driverButton1"(FALSE ("driverButton1")) -> (error out=w339:errorcluster)  [unwired: 1 in]
            n163 = shared-variable ".\\Shared Variables.lvlib\\Driver.lvlib\\driverButton6"(FALSE ("driverButton1"), error in=w339) -> (error out=w343:errorcluster)
            n164 = shared-variable ".\\Shared Variables.lvlib\\Driver.lvlib\\driverButton8"(TRUE ("driverButton1"), error in=w343) -> ()  [unwired: 1 out]
          }
          frame 23 {
            # "wait for fire"
            n165 = Increment(x=w349) -> (x+1=w352:i32)
            n166 = call "Delay.vi"("Timer Going?"=TRUE, "Time to Wait (ms)"=350.0) -> ("Time Up"=w351:bool)
            n167 = Select(t=w352, s=w351, f=w349) -> (s? t:f=w348:i32)
          }
          frame 24 {
            # "stop fire\nretract arm"
            n168 = shared-variable ".\\Shared Variables.lvlib\\Driver.lvlib\\driverButton8"(FALSE ("driverButton8")) -> (error out=w356:errorcluster)  [unwired: 1 in]
            n169 = shared-variable ".\\Shared Variables.lvlib\\Driver.lvlib\\driverButton7"(TRUE ("driverButton8"), error in=w356) -> ()  [unwired: 1 out]
            n170 = Increment(x=w358) -> (x+1=w357:i32)
          }
          frame 25 {
            # "wait for retract"
            n171 = call <vilib>:"WPI_AnalogChannelGetVoltage.vi"("AIDeviceRef"=w363) -> ("Voltage"=w367:dbl)  [unwired: 8 in, 2 out]
            n172 = In Range and Coerce(upper limit=5.0, x=w367, lower limit=1.5) -> (In Range?=w364:bool)  [unwired: 1 out]
            n173 = Increment(x=w368) -> (x+1=w370:i32)
            n174 = Select(t=w370, s=w364, f=w368) -> (s? t:f=w369:i32)
          }
          frame 26 {
            # "bring intake arm up\nEND AUTO"
            n175 = shared-variable ".\\Shared Variables.lvlib\\Driver.lvlib\\driverButton7"(FALSE ("driverButton8")) -> (error out=w374:errorcluster)  [unwired: 1 in]
            n176 = shared-variable ".\\Shared Variables.lvlib\\Driver.lvlib\\driverButton1"(TRUE ("driverButton1"), error in=w374) -> ()  [unwired: 1 out]
          }
          frame 29 {
            n177 = shared-variable ".\\Shared Variables.lvlib\\Driver.lvlib\\driverJoystickAxis1"(0.0 ("driverJoystickAxis1")) -> ()  [unwired: 1 in, 1 out]
          }
        }
        n178 = Select(t=cluster{"output high":dbl, "output low":dbl} {"output high"=0.0, "output low"=0.0} ("output range"), s=w126, f=cluster{"output high":dbl, "output low":dbl} {"output high"=0.6, "output low"=-0.6} ("output range")) -> (s? t:f=w127:cluster{"output high":dbl, "output low":dbl})
        n179 = call-poly <vilib>:"PID.vi"("reinitialize? (F)"=w126, "output range"=w127, "PID gains"=w133, "process variable"=w125, "setpoint"=w134) -> ("output"=w138:dbl)  [unwired: 5 in, 1 out]
        n180 = shared-variable ".\\Shared Variables.lvlib\\Driver.lvlib\\driverJoystickAxis3"(w138) -> ()  [unwired: 1 in, 1 out]
        "State 2" <- w136
      }
    }
    frame 16 {
      n181 = call <vilib>:"WPI_EncoderRefNum Registry Get.vi"("refnum name"="leftWheelEncoder") -> ("EncoderDevRef"=w402:T3)  [unwired: 9 in, 1 out]
      n182 = call <vilib>:"WPI_EncoderRefNum Registry Get.vi"("refnum name"="rightWheelEncoder") -> ("EncoderDevRef"=w401:T3)  [unwired: 9 in, 1 out]
      n183 = call <vilib>:"WPI_GyroRefNum Registry Get.vi"("refnum name"="yawGyro") -> ("error out"=w389:errorcluster, "GyroDevRef"=w390:T7)  [unwired: 9 in]
      n184 = call <vilib>:"WPI_GyroReset.vi"("error in (no error)"=w389, "GyroDevRef"=w390) -> ("GyroDevRef"=w387:T7)  [unwired: 8 in, 1 out]
      n185 = call <vilib>:"WPI_EncoderReset.vi"("EncoderDevRef"=w402) -> ("EncoderDevRef"=w397:T3)  [unwired: 9 in, 1 out]
      n186 = call <vilib>:"WPI_EncoderReset.vi"("EncoderDevRef"=w401) -> ("EncoderDevRef"=w396:T3)  [unwired: 9 in, 1 out]
      n187 = call <vilib>:"WPI_AnalogChannelRefNum Registry Get.vi"("refnum name"="irProximDistCatapult") -> ("AIDeviceRef"=w395:T10)  [unwired: 9 in, 1 out]
      n188 = call <vilib>:"WPI_AnalogChannelRefNum Registry Get.vi"("refnum name"="irProximDistCatDown") -> ("AIDeviceRef"=w391:T10)  [unwired: 9 in, 1 out]
      n189 = Get Date/Time In Seconds() -> (seconds since 1Jan1904=w383:timestamp)
      n190 = call <vilib>:"WPI_DigitalInputRefNum Registry Get.vi"("refnum name"="irProximSwitchLeftIntake") -> ("DigitalInputDevRef"=w384:T11)  [unwired: 9 in, 1 out]
      n191 = while {
        tunnel: w398 -> [w437]
        tunnel: w397 -> [w436]
        tunnel: w396 -> [w435]
        tunnel: w395 -> [w411]
        shift-right: [w429] -> _
        shift-left: 0 -> [w432]
        tunnel: w391 -> [w410]
        tunnel: w387 -> [_]
        tunnel: w386 -> [w430]
        tunnel: w383 -> [w427]
        tunnel: w384 -> [w419]
        shift-right: [w409] -> _
        shift-left: w383 -> [w408]
        tunnel: w382 -> [w405]
        tunnel: w381 -> [w404]
        stop <- FALSE stop-if-true
        n192 = shared-variable ".\\Shared Variables.lvlib\\Sensors-Actuators.lvlib\\Gyro.lvlib\\yawGyro"() -> (w422:dbl)  [unwired: 1 in, 1 out]
        "Waveform Chart 2" <- w422
        n193 = call <vilib>:"WPI_DigitalInputGetValue.vi"("DigitalInputDevRef"=w419) -> ("Value"=w420:bool)  [unwired: 8 in, 2 out]
        n194 = Wait (ms)(milliseconds to wait=u32 25) -> ()  [unwired: 1 out]
        n195 = call <vilib>:"WPI_AnalogChannelGetVoltage.vi"("AIDeviceRef"=w410) -> ("Voltage"=w412:dbl)  [unwired: 8 in, 2 out]
        n196 = Not(x=w420) -> (.not. x?=w418:bool)
        n197 = call-poly <vilib>:"PID Control Input Filter.vi"("input"=w412) -> ("output"=w421:dbl)  [unwired: 4 in]
        n198 = Boolean To (0,1)(Boolean=w418) -> (0, 1=w414:i16)
        n199 = call-poly <vilib>:"PID Control Input Filter.vi"("input"=w414) -> ("output"=w417:dbl)  [unwired: 4 in]
        n200 = call <userlib>:"Schmitt Trigger.vi"("lo"=sgl 0.1 ("High to Low\nTransition"), "in"=w417, "hi"=sgl 0.9 ("Low to High\nTransition")) -> ("out"=w413:bool)  [unwired: 1 out]
        n201 = case shown="13" w432 {
          selector: w432 -> [_ w455 w472 w493 w508 w531 w548 w563 w576 w592 w618 w633 w645 w652 w664 w674 w683 w688 w697 w712 w721 w732 w736]
          tunnel: [4 ("t") w457 w484 w492 w507 w537 w551 w562 w575 w591 w616 w631 w644 w651 w663 w673 w682 w687 w699 w711 w720 w733 w736] -> w429
          tunnel: w437 -> [_ _ w487 _ _ _ _ _ _ _ w596 _ _ _ _ _ _ _ _ _ _ _ _]
          tunnel: w436 -> [_ _ w486 _ w506 _ _ _ _ w580 w610 _ _ _ _ _ _ _ _ _ _ _ _]
          tunnel: w435 -> [_ _ w485 _ w505 _ _ _ _ w581 w609 _ _ _ _ _ _ _ _ _ _ _ _]
          tunnel: w410 -> [_ _ _ _ _ _ _ _ _ w590 _ _ _ _ _ _ _ _ _ _ _ w727 _]
          tunnel: [0.0 ("setpoint") 0.0 ("setpoint") 0.0 ("setpoint") 0.0 ("setpoint") 0.0 ("setpoint") w535 w550 w568 w574 w585 w622 w630 w641 w650 w662 w672 w681 w686 w701 w710 w718 w726 w738] -> w431
          tunnel: w422 -> [_ _ _ _ _ w536 w550 w568 w574 w585 w622 w630 w641 w650 w662 w672 w681 w686 w701 w710 w718 w726 w738]
          tunnel: [FALSE FALSE FALSE FALSE FALSE FALSE TRUE TRUE TRUE TRUE TRUE TRUE TRUE TRUE TRUE TRUE TRUE TRUE TRUE TRUE TRUE TRUE TRUE] -> w423
          tunnel: w427 -> [w440 w451 w460 w488 _ _ w542 w561 w571 w579 w603 w626 w639 w647 w656 w668 w678 w684 w694 w708 w716 w724 w735]
          tunnel: w421 -> [_ _ _ _ _ _ _ w564 _ _ _ _ _ _ _ _ _ _ w696 _ _ _ _]
          tunnel: w413 -> [_ _ _ _ _ _ _ _ _ _ w615 _ _ _ _ _ _ _ _ _ _ _ _]
          tunnel: w411 -> [_ _ _ _ _ _ _ _ _ _ _ w628 _ _ _ _ _ _ _ _ _ _ _]
          tunnel: [w440 w451 w460 w488 w498 w517 w542 w561 w571 w579 w603 w626 w639 w647 w656 w668 w678 w684 w694 w708 w716 w724 w735] -> w409
          tunnel: w408 -> [_ _ _ _ _ w517 _ _ _ _ _ _ _ _ _ _ _ _ _ _ _ _ _]
          tunnel: "Catapult Down" -> [_ _ _ _ _ _ _ w560 _ _ _ _ _ _ _ _ _ _ w693 _ _ _ _]
          tunnel: "Fire Delay" -> [_ _ _ _ _ _ _ _ w570 _ _ _ _ _ _ _ _ _ _ w707 _ _ _]
          tunnel: w405 -> [_ _ _ _ _ w515 _ _ _ _ _ _ _ _ _ _ _ _ _ _ _ _ _]
          tunnel: w404 -> [_ _ _ _ _ _ _ _ _ _ _ _ _ _ _ _ _ _ _ _ _ _ _]
          frame 0, Default {
            # "switch to manual\nSet intake speed to slow\nLower intake\nStart intake motor"
            n202 = shared-variable ".\\Shared Variables.lvlib\\Driver.lvlib\\driverButton10"(TRUE ("driverButton10")) -> (error out=w442:errorcluster)  [unwired: 1 in]
            n203 = shared-variable ".\\Shared Variables.lvlib\\Misc..lvlib\\Desired Intake Speed"(0.2 ("Intake RPM"), error in=w442) -> (error out=w441:errorcluster)
            n204 = shared-variable ".\\Shared Variables.lvlib\\Driver.lvlib\\driverButton6"(TRUE ("driverButton6"), error in=w441) -> (error out=w444:errorcluster)
            n205 = shared-variable ".\\Shared Variables.lvlib\\Driver.lvlib\\driverButton1"(TRUE ("driverButton1"), error in=w444) -> (error out=w438:errorcluster)
            n206 = shared-variable ".\\Shared Variables.lvlib\\Driver.lvlib\\driverButton7"(FALSE ("driverButton8"), error in=w438) -> ()  [unwired: 1 out]
          }
          frame 4 {
            # "wait for intake to lower"
            n207 = call "Delay.vi"("Timer Going?"=TRUE, "Time to Wait (ms)"=450.0) -> ("Time Up"=w458:bool)
            n208 = Select(t=7, s=w458, f=w455) -> (s? t:f=w457:i32)
          }
          frame 7 {
            # "turn intake off\nset intake speed to ful"
            # "run intake\ndrive"
            n209 = call <vilib>:"WPI_EncoderGet.vi"("EncoderDevRef"=w486) -> ("Distance"=w478:dbl)  [unwired: 5 in, 5 out]
            n210 = call <vilib>:"WPI_EncoderGet.vi"("EncoderDevRef"=w485) -> ("Distance"=w477:dbl)  [unwired: 5 in, 5 out]
            n211 = Add(x=w478, y=w477) -> (x+y=w476:dbl)
            n212 = Divide(x=w476, y=2.0) -> (x/y=w474:dbl)
            n213 = Divide(x=250.0, y=360.0) -> (x/y=w481:dbl)
            n214 = Multiply(x="auto 3 distance 5", y=w481) -> (x*y=w483:dbl)
            n215 = Select(t=w483, s=w487, f="auto 3 distance 5") -> (s? t:f=w473:dbl)
            n216 = Greater?(x=w474, y=w473) -> (0:w462:bool)
            n217 = Select(t=0.0, s=w462, f=-0.8 ("driverJoystickAxis2")) -> (s? t:f=w463:dbl)
            n218 = Select(t=3, s=w462, f=w472) -> (s? t:f=w484:i32)
            n219 = shared-variable ".\\Shared Variables.lvlib\\Driver.lvlib\\driverJoystickAxis2"(w463) -> (error out=w461:errorcluster)  [unwired: 1 in]
            n220 = shared-variable ".\\Shared Variables.lvlib\\Driver.lvlib\\driverButton6"(TRUE ("driverButton6")) -> ()  [unwired: 1 in, 1 out]
            n221 = shared-variable ".\\Shared Variables.lvlib\\Misc..lvlib\\Desired Intake Speed"(1.0 ("Desired Intake Speed"), error in=w461) -> ()  [unwired: 1 out]
            n222 = shared-variable ".\\Shared Variables.lvlib\\Driver.lvlib\\driverButton1"(FALSE ("driverButton1")) -> ()  [unwired: 1 in, 1 out]
          }
          frame 3 {
            # "Wait 300ms after stoping"
            n223 = call "Delay.vi"("Timer Going?"=TRUE, "Time to Wait (ms)"=300.0) -> ("Time Up"=w495:bool)
            n224 = Select(t=9 ("x"), s=w495, f=w493) -> (s? t:f=w492:i32)
          }
          frame 9 {
            # "wait for encoder to stop"
            n225 = call <vilib>:"WPI_EncoderGet.vi"("EncoderDevRef"=w506) -> ("Stopped"=w504:bool)  [unwired: 5 in, 5 out]
            n226 = call <vilib>:"WPI_EncoderGet.vi"("EncoderDevRef"=w505) -> ("Stopped"=w503:bool)  [unwired: 5 in, 5 out]
            n227 = And(x=w504, y=w503) -> (x .and. y?=w502:bool)
            n228 = Select(t=32, s=w502, f=w508) -> (s? t:f=w507:i32)
            n229 = shared-variable ".\\Shared Variables.lvlib\\Driver.lvlib\\driverButton6"(FALSE ("driverButton6")) -> ()  [unwired: 1 in, 1 out]
            n230 = Get Date/Time In Seconds() -> (seconds since 1Jan1904=w498:timestamp)
          }
          frame 32 {
            w527 = 1.0 ("f")
            # "Turn robot X degrees"
            n231 = To Double Precision Float(number=w517) -> (double precision float=w521:dbl)
            n232 = Get Date/Time In Seconds() -> (seconds since 1Jan1904=w523:timestamp)
            n233 = shared-variable ".\\Shared Variables.lvlib\\Driver.lvlib\\driverButton6"(FALSE ("driverButton6")) -> ()  [unwired: 1 in, 1 out]
            n234 = shared-variable ".\\Shared Variables.lvlib\\Driver.lvlib\\driverJoystickAxis2"(0.0 ("driverJoystickAxis2")) -> ()  [unwired: 1 in, 1 out]
            n235 = To Double Precision Float(number=w523) -> (double precision float=w522:dbl)
            n236 = Add(x=w521, y="Abort Turn") -> (x+y=w525:dbl)
            n237 = shared-variable ".\\Shared Variables.lvlib\\Dashboard Variables.lvlib\\Kinect Status"() -> (w516:bool)  [unwired: 1 in, 1 out]
            "Turn Left 2" <- w516
            n238 = Or(x=w516, y=w515) -> (x .or. y?=w514:bool)
            n239 = Less?(x=w525, y=w522) -> (x < y?=w520:bool)
            n240 = Select(t="Left Rotate", s=w514, f=0.0) -> (s? t:f=w512:dbl)
            n241 = Negate(x=w527) -> ()  [unwired: 1 out]
            n242 = Select(t="left turn angle 3", s=w514, f="right turn angle 3") -> (s? t:f=w535:dbl)
            n243 = Select(t="Left Strafe", s=w514, f=w527) -> (s? t:f=w528:dbl)
            n244 = disable-structure shown="Disabled" {
              frame Disabled {
                n245 = shared-variable ".\\Shared Variables.lvlib\\Driver.lvlib\\driverJoystickAxis1"(0.0 ("driverJoystickAxis1")) -> ()  [unwired: 1 in, 1 out]
              }
              frame Enabled {
              }
            }
            n246 = shared-variable ".\\Shared Variables.lvlib\\Driver.lvlib\\driverJoystickAxis1"(w528) -> ()  [unwired: 1 in, 1 out]
            n247 = Subtract(x=w536, y=w535) -> (x-y=w534:dbl)
            n248 = shared-variable ".\\Shared Variables.lvlib\\Driver.lvlib\\driverJoystickAxis3"(w512) -> ()  [unwired: 1 in, 1 out]
            n249 = Absolute Value(x=w534) -> (abs(x)=w533:dbl)
            n250 = Less Or Equal?(x=w533, y=3.0) -> (x <= y?=w519:bool)
            n251 = Or(x=w519, y=w520) -> (x .or. y?=w518:bool)
            n252 = Select(t=33, s=w518, f=w531) -> (s? t:f=w537:i32)
          }
          frame 33 {
            w541 = 0.0 ("driverJoystickAxis1")
            # "This loop is for settling down after turning the robot.\nIncrease this loop to ensure Ball 1 goes through in \n2nd 5-second period."
            # "Wait for settling after turn"
            n253 = shared-variable ".\\Shared Variables.lvlib\\Driver.lvlib\\driverJoystickAxis1"(0.0 ("driverJoystickAxis1")) -> ()  [unwired: 1 in, 1 out]
            n254 = To Double Precision Float(number=w542) -> (double precision float=w543:dbl)
            n255 = shared-variable ".\\Shared Variables.lvlib\\Driver.lvlib\\driverJoystickAxis3"(w541) -> ()  [unwired: 1 in, 1 out]
            n256 = shared-variable ".\\Shared Variables.lvlib\\Driver.lvlib\\driverJoystickAxis1"(w541) -> ()  [unwired: 1 in, 1 out]
            n257 = while {
              tunnel: w543 -> [w553]
              stop <- w556 continue-if-true
              n258 = Wait (ms)(milliseconds to wait=u32 10) -> ()  [unwired: 1 out]
              n259 = Get Date/Time In Seconds() -> (seconds since 1Jan1904=w559:timestamp)
              n260 = To Double Precision Float(number=w559) -> (double precision float=w557:dbl)
              n261 = Add(x=w553, y="When To Start Firing 2") -> (x+y=w558:dbl)
              n262 = Greater?(x=w558, y=w557) -> (0:w556:bool)
            }
            n263 = shared-variable ".\\Shared Variables.lvlib\\Driver.lvlib\\driverJoystickAxis2"(w541) -> ()  [unwired: 1 in, 1 out]
            n264 = call "Delay.vi"("Timer Going?"=TRUE, "Time to Wait (ms)"=250.0) -> ("Time Up"=w545:bool)
            n265 = Select(t=10, s=w545, f=w548) -> (s? t:f=w551:i32)
          }
          frame 10 {
            # "Combine states 10 & 11"
            # "Fire 1"
            # "fire"
            n266 = Increment(x=w563) -> (x+1=w566:i32)
            n267 = Greater Or Equal?(x=w560, y=w564) -> (x >= y?=w565:bool)
            n268 = shared-variable ".\\Shared Variables.lvlib\\Driver.lvlib\\driverButton8"(TRUE ("driverButton8")) -> ()  [unwired: 1 in, 1 out]
            n269 = Select(t=w566, s=w565, f=w563) -> (s? t:f=w562:i32)
          }
          frame 11 {
            # "wait for fire to comlete"
            n270 = call "Delay.vi"("Timer Going?"=TRUE, "Time to Wait (ms)"=w570) -> ("Time Up"=w577:bool)
            n271 = Select(t=13, s=w577, f=w576) -> (s? t:f=w575:i32)
          }
          frame 13 {
            # "wait for arm to come down"
            n272 = call <vilib>:"WPI_EncoderReset.vi"("EncoderDevRef"=w581) -> ()  [unwired: 9 in, 2 out]
            n273 = call <vilib>:"WPI_AnalogChannelGetVoltage.vi"("AIDeviceRef"=w590) -> ("Voltage"=w589:dbl)  [unwired: 8 in, 2 out]
            n274 = Increment(x=w592) -> (x+1=w593:i32)
            n275 = shared-variable ".\\Shared Variables.lvlib\\Driver.lvlib\\driverButton8"(FALSE ("driverButton8")) -> ()  [unwired: 1 in, 1 out]
            n276 = shared-variable ".\\Shared Variables.lvlib\\Driver.lvlib\\driverButton7"(TRUE ("driverButton8")) -> ()  [unwired: 1 in, 1 out]
            n277 = call <vilib>:"WPI_EncoderReset.vi"("EncoderDevRef"=w580) -> ()  [unwired: 9 in, 2 out]
            n278 = In Range and Coerce(upper limit=5.0, x=w589, lower limit=1.8) -> (In Range?=w586:bool)  [unwired: 1 out]
            n279 = Select(t=w593, s=w586, f=w592) -> (s? t:f=w591:i32)
          }
          frame 14 {
            # "intake ball 2"
            n280 = call <vilib>:"WPI_EncoderGet.vi"("EncoderDevRef"=w609) -> ("Distance"=w613:dbl)  [unwired: 5 in, 5 out]
            n281 = call <vilib>:"WPI_EncoderGet.vi"("EncoderDevRef"=w610) -> ("Distance"=w614:dbl)  [unwired: 5 in, 5 out]
            n282 = Increment(x=w618) -> (x+1=w617:i32)
            n283 = Add(x=w614, y=w613) -> (x+y=w612:dbl)
            n284 = shared-variable ".\\Shared Variables.lvlib\\Driver.lvlib\\driverButton7"(FALSE ("driverButton8")) -> (error out=w623:errorcluster)  [unwired: 1 in]
            n285 = Divide(x=w612, y=2.0) -> (x/y=w602:dbl)
            n286 = Absolute Value(x=w602) -> (abs(x)=w601:dbl)
            n287 = Divide(x=250.0, y=360.0) -> (x/y=w598:dbl)
            n288 = shared-variable ".\\Shared Variables.lvlib\\Driver.lvlib\\driverButton6"(TRUE ("driverButton1"), error in=w623) -> (error out=w619:errorcluster)
            n289 = Multiply(x="BackupLimit", y=w598) -> (x*y=w600:dbl)
            n290 = Select(t=w600, s=w596, f="BackupLimit") -> (s? t:f=w594:dbl)
            n291 = Greater Or Equal?(x=w601, y=w594) -> (x >= y?=w608:bool)
            n292 = Or(x=w608, y=w615) -> (x .or. y?=w607:bool)
            n293 = Select(t=w617, s=w607, f=w618) -> (s? t:f=w616:i32)
            n294 = Select(t=0.0, s=w607, f="BackupSpeed") -> (s? t:f=w604:dbl)
            n295 = shared-variable ".\\Shared Variables.lvlib\\Driver.lvlib\\driverJoystickAxis2"(w604) -> ()  [unwired: 1 in, 1 out]
            n296 = shared-variable ".\\Shared Variables.lvlib\\Misc..lvlib\\Desired Intake Speed"(1.0 ("Desired Intake Speed"), error in=w619) -> ()  [unwired: 1 out]
          }
          frame 15 {
            # "Consider decreasing settling time"
            # "wait for intake to finish"
            n297 = call <vilib>:"WPI_AnalogChannelGetVoltage.vi"("AIDeviceRef"=w628) -> ("Voltage"=w627:dbl)  [unwired: 8 in, 2 out]
            n298 = In Range and Coerce(upper limit=5.0, x=w627, lower limit=0.6) -> (In Range?=w636:bool)  [unwired: 1 out]
            n299 = call "Stable.vi"("Eval Period (sec)"=0.03, "Signal Input"=w636) -> ("Stable"=w634:bool)  [unwired: 9 in]
            n300 = Increment(x=w633) -> (x+1=w632:i32)
            n301 = Select(t=w632, s=w634, f=w633) -> (s? t:f=w631:i32)
          }
          frame 16 {
            # "raise intake\nstop intaking"
            n302 = shared-variable ".\\Shared Variables.lvlib\\Driver.lvlib\\driverButton6"(FALSE ("driverButton1")) -> (error out=w642:errorcluster)  [unwired: 1 in]
            n303 = shared-variable ".\\Shared Variables.lvlib\\Driver.lvlib\\driverButton1"(TRUE ("driverButton1"), error in=w642) -> ()  [unwired: 1 out]
            n304 = Increment(x=w645) -> (x+1=w644:i32)
          }
          frame 17 {
            # "wait for intake to raise\nDelay for CMD"
            n305 = call "Delay.vi"("Timer Going?"=TRUE, "Time to Wait (ms)"=100.0) -> ("Time Up"=w654:bool)
            n306 = Select(t=27, s=w654, f=w652) -> (s? t:f=w651:i32)
          }
          frame 27 {
            # "wait for intake to raise\nDelay for CMD"
            n307 = shared-variable ".\\Shared Variables.lvlib\\Driver.lvlib\\driverButton1"(FALSE ("driverButton1")) -> (error out=w657:errorcluster)  [unwired: 1 in]
            n308 = shared-variable ".\\Shared Variables.lvlib\\Misc..lvlib\\Desired Intake Speed"(0.2 ("Desired Intake Speed"), error in=w657) -> ()  [unwired: 1 out]
            n309 = call "Delay.vi"("Timer Going?"=TRUE, "Time to Wait (ms)"=100.0) -> ("Time Up"=w666:bool)
            n310 = Select(t=28, s=w666, f=w664) -> (s? t:f=w663:i32)
          }
          frame 28 {
            # "Typically 250ms"
            # "wait for intake to raise\nDelay for CMD"
            n311 = shared-variable ".\\Shared Variables.lvlib\\Driver.lvlib\\driverButton6"(TRUE ("driverButton1")) -> ()  [unwired: 1 in, 1 out]
            n312 = call "Delay.vi"("Timer Going?"=TRUE, "Time to Wait (ms)"=500.0) -> ("Time Up"=w676:bool)
            n313 = Select(t=20, s=w676, f=w674) -> (s? t:f=w673:i32)
          }
          frame 20 {
            # "run intake motor\n lower intake"
            n314 = Increment(x=w683) -> (x+1=w682:i32)
            n315 = shared-variable ".\\Shared Variables.lvlib\\Driver.lvlib\\driverButton1"(TRUE ("driverButton1")) -> ()  [unwired: 1 in, 1 out]
          }
          frame 21 {
            # "Consider decreasing settling time"
            # "wait for intake to lower\n(450ms)"
            n316 = Increment(x=w688) -> (x+1=w691:i32)
            n317 = call "Delay.vi"("Timer Going?"=TRUE, "Time to Wait (ms)"=450.0 ("Wait for Intake to Lower (450ms)")) -> ("Time Up"=w690:bool)
            n318 = Select(t=w691, s=w690, f=w688) -> (s? t:f=w687:i32)
          }
          frame 22 {
            # "stop running intake motor\nfire\nDe-Assert Lower Intake"
            n319 = Increment(x=w697) -> (x+1=w698:i32)
            n320 = Greater Or Equal?(x=w693, y=w696) -> (x >= y?=w695:bool)
            n321 = Select(t=w698, s=w695, f=w697) -> (s? t:f=w699:i32)
            n322 = shared-variable ".\\Shared Variables.lvlib\\Driver.lvlib\\driverButton1"(FALSE ("driverButton1")) -> (error out=w702:errorcluster)  [unwired: 1 in]
            n323 = shared-variable ".\\Shared Variables.lvlib\\Driver.lvlib\\driverButton6"(FALSE ("driverButton1"), error in=w702) -> (error out=w704:errorcluster)
            n324 = shared-variable ".\\Shared Variables.lvlib\\Driver.lvlib\\driverButton8"(TRUE ("driverButton1"), error in=w704) -> ()  [unwired: 1 out]
          }
          frame 23 {
            # "wait for fire"
            n325 = Increment(x=w712) -> (x+1=w715:i32)
            n326 = call "Delay.vi"("Timer Going?"=TRUE, "Time to Wait (ms)"=w707) -> ("Time Up"=w714:bool)
            n327 = Select(t=w715, s=w714, f=w712) -> (s? t:f=w711:i32)
          }
          frame 24 {
            # "stop fire\nretract arm"
            n328 = shared-variable ".\\Shared Variables.lvlib\\Driver.lvlib\\driverButton8"(FALSE ("driverButton8")) -> (error out=w719:errorcluster)  [unwired: 1 in]
            n329 = shared-variable ".\\Shared Variables.lvlib\\Driver.lvlib\\driverButton7"(TRUE ("driverButton8"), error in=w719) -> ()  [unwired: 1 out]
            n330 = Increment(x=w721) -> (x+1=w720:i32)
          }
          frame 25 {
            # "wait for retract"
            n331 = call <vilib>:"WPI_AnalogChannelGetVoltage.vi"("AIDeviceRef"=w727) -> ("Voltage"=w731:dbl)  [unwired: 8 in, 2 out]
            n332 = In Range and Coerce(upper limit=5.0, x=w731, lower limit=1.5) -> (In Range?=w728:bool)  [unwired: 1 out]
            n333 = Increment(x=w732) -> (x+1=w734:i32)
            n334 = Select(t=w734, s=w728, f=w732) -> (s? t:f=w733:i32)
          }
          frame 26 {
            # "bring intake arm up\nEND AUTO"
            n335 = shared-variable ".\\Shared Variables.lvlib\\Driver.lvlib\\driverButton7"(FALSE ("driverButton8")) -> (error out=w739:errorcluster)  [unwired: 1 in]
            n336 = shared-variable ".\\Shared Variables.lvlib\\Driver.lvlib\\driverButton1"(TRUE ("driverButton1"), error in=w739) -> ()  [unwired: 1 out]
          }
        }
        n337 = Select(t=cluster{"output high":dbl, "output low":dbl} {"output high"=0.0, "output low"=0.0} ("output range"), s=w423, f=cluster{"output high":dbl, "output low":dbl} {"output high"=0.6, "output low"=-0.6} ("output range")) -> (s? t:f=w424:cluster{"output high":dbl, "output low":dbl})
        n338 = call-poly <vilib>:"PID.vi"("reinitialize? (F)"=w423, "output range"=w424, "PID gains"=w430, "process variable"=w422, "setpoint"=w431) -> ("output"=w433:dbl)  [unwired: 5 in, 1 out]
        n339 = shared-variable ".\\Shared Variables.lvlib\\Driver.lvlib\\driverJoystickAxis3"(w433) -> ()  [unwired: 1 in, 1 out]
        "State 3" <- w432
      }
    }
    frame 32 {
      n340 = call <vilib>:"WPI_EncoderRefNum Registry Get.vi"("refnum name"="leftWheelEncoder") -> ("EncoderDevRef"=w763:T3)  [unwired: 9 in, 1 out]
      n341 = call <vilib>:"WPI_EncoderRefNum Registry Get.vi"("refnum name"="rightWheelEncoder") -> ("EncoderDevRef"=w762:T3)  [unwired: 9 in, 1 out]
      n342 = call <vilib>:"WPI_GyroRefNum Registry Get.vi"("refnum name"="yawGyro") -> ("error out"=w750:errorcluster, "GyroDevRef"=w751:T7)  [unwired: 9 in]
      n343 = call <vilib>:"WPI_GyroReset.vi"("error in (no error)"=w750, "GyroDevRef"=w751) -> ("GyroDevRef"=w748:T7)  [unwired: 8 in, 1 out]
      n344 = call <vilib>:"WPI_EncoderReset.vi"("EncoderDevRef"=w763) -> ("EncoderDevRef"=w758:T3)  [unwired: 9 in, 1 out]
      n345 = call <vilib>:"WPI_EncoderReset.vi"("EncoderDevRef"=w762) -> ("EncoderDevRef"=w757:T3)  [unwired: 9 in, 1 out]
      n346 = call <vilib>:"WPI_AnalogChannelRefNum Registry Get.vi"("refnum name"="irProximDistCatapult") -> ("AIDeviceRef"=w756:T10)  [unwired: 9 in, 1 out]
      n347 = call <vilib>:"WPI_AnalogChannelRefNum Registry Get.vi"("refnum name"="irProximDistCatDown") -> ("AIDeviceRef"=w752:T10)  [unwired: 9 in, 1 out]
      n348 = Get Date/Time In Seconds() -> (seconds since 1Jan1904=w744:timestamp)
      n349 = call <vilib>:"WPI_DigitalInputRefNum Registry Get.vi"("refnum name"="irProximSwitchLeftIntake") -> ("DigitalInputDevRef"=w745:T11)  [unwired: 9 in, 1 out]
      n350 = while {
        tunnel: w759 -> [w798]
        tunnel: w758 -> [w797]
        tunnel: w757 -> [w796]
        tunnel: w756 -> [w772]
        shift-right: [w790] -> _
        shift-left: 0 -> [w793]
        tunnel: w752 -> [w771]
        tunnel: w748 -> [_]
        tunnel: w747 -> [w791]
        tunnel: w744 -> [w788]
        tunnel: w745 -> [w780]
        shift-right: [w770] -> _
        shift-left: w744 -> [w769]
        tunnel: w743 -> [w766]
        tunnel: w742 -> [w765]
        stop <- FALSE stop-if-true
        n351 = shared-variable ".\\Shared Variables.lvlib\\Sensors-Actuators.lvlib\\Gyro.lvlib\\yawGyro"() -> (w783:dbl)  [unwired: 1 in, 1 out]
        "Waveform Chart 3" <- w783
        n352 = call <vilib>:"WPI_DigitalInputGetValue.vi"("DigitalInputDevRef"=w780) -> ("Value"=w781:bool)  [unwired: 8 in, 2 out]
        n353 = Wait (ms)(milliseconds to wait=u32 25) -> ()  [unwired: 1 out]
        n354 = call <vilib>:"WPI_AnalogChannelGetVoltage.vi"("AIDeviceRef"=w771) -> ("Voltage"=w773:dbl)  [unwired: 8 in, 2 out]
        n355 = Not(x=w781) -> (.not. x?=w779:bool)
        n356 = call-poly <vilib>:"PID Control Input Filter.vi"("input"=w773) -> ("output"=w782:dbl)  [unwired: 4 in]
        n357 = Boolean To (0,1)(Boolean=w779) -> (0, 1=w775:i16)
        n358 = call-poly <vilib>:"PID Control Input Filter.vi"("input"=w775) -> ("output"=w778:dbl)  [unwired: 4 in]
        n359 = call <userlib>:"Schmitt Trigger.vi"("lo"=sgl 0.1 ("High to Low\nTransition"), "in"=w778, "hi"=sgl 0.9 ("Low to High\nTransition")) -> ("out"=w774:bool)  [unwired: 1 out]
        n360 = case shown="10" w793 {
          selector: w793 -> [_ w816 w857 w879 w894 w923 w938 w953 w966 w982 w1008 w1023 w1035 w1042 w1054 w1064 w1073 w1078 w1087 w1102 w1111 w1122 w1126 w1144]
          tunnel: [4 ("t") w818 w866 w878 w893 w927 w941 w952 w965 w981 w1006 w1021 w1034 w1041 w1053 w1063 w1072 w1077 w1089 w1101 w1110 w1123 w1125 w1144] -> w790
          tunnel: w798 -> [_ _ w831 _ _ _ _ _ _ _ w986 _ _ _ _ _ _ _ _ _ _ _ _ _]
          tunnel: w797 -> [_ _ w868 _ w892 _ _ _ _ w970 w1000 _ _ _ _ _ _ _ _ _ _ _ _ _]
          tunnel: w796 -> [_ _ w867 _ w891 _ _ _ _ w971 w999 _ _ _ _ _ _ _ _ _ _ _ _ _]
          tunnel: w771 -> [_ _ _ _ _ _ _ _ _ w980 _ _ _ _ _ _ _ _ _ _ _ w1117 _ _]
          tunnel: [0.0 ("setpoint") 0.0 ("setpoint") 0.0 ("setpoint") 0.0 ("setpoint") 0.0 ("setpoint") w898 w940 w958 w964 w975 w1012 w1020 w1031 w1040 w1052 w1062 w1071 w1076 w1091 w1100 w1108 w1116 w1133 w1143] -> w792
          tunnel: w783 -> [_ _ _ _ _ w901 w940 w958 w964 w975 w1012 w1020 w1031 w1040 w1052 w1062 w1071 w1076 w1091 w1100 w1108 w1116 w1133 w1143]
          tunnel: [FALSE FALSE FALSE FALSE FALSE FALSE TRUE TRUE TRUE TRUE TRUE TRUE TRUE TRUE TRUE TRUE TRUE TRUE TRUE TRUE TRUE TRUE TRUE TRUE] -> w784
          tunnel: w788 -> [w801 w812 _ w874 _ _ w932 w951 w961 w969 w993 w1016 w1029 w1037 w1046 w1058 w1068 w1074 w1084 w1098 w1106 w1114 w1131 w1141]
          tunnel: w782 -> [_ _ _ _ _ _ _ w954 _ _ _ _ _ _ _ _ _ _ w1086 _ _ _ _ _]
          tunnel: w774 -> [_ _ _ _ _ _ _ _ _ _ w1005 _ _ _ _ _ _ _ _ _ _ _ _ _]
          tunnel: w772 -> [_ _ _ _ _ _ _ _ _ _ _ w1018 _ _ _ _ _ _ _ _ _ _ _ _]
          tunnel: [w801 w812 w821 w874 w884 w910 w932 w951 w961 w969 w993 w1016 w1029 w1037 w1046 w1058 w1068 w1074 w1084 w1098 w1106 w1114 w1131 w1141] -> w770
          tunnel: w769 -> [_ _ _ _ _ w910 _ _ _ _ _ _ _ _ _ _ _ _ _ _ _ _ _ _]
          tunnel: "Catapult Down 2" -> [_ _ _ _ _ _ _ w950 _ _ _ _ _ _ _ _ _ _ w1083 _ _ _ _ _]
          tunnel: "Fire Delay 2" -> [_ _ _ _ _ _ _ _ w960 _ _ _ _ _ _ _ _ _ _ w1097 _ _ _ _]
          tunnel: w766 -> [_ _ _ _ _ w908 _ _ _ _ _ _ _ _ _ _ _ _ _ _ _ _ _ _]
          tunnel: w765 -> [_ _ _ _ _ _ _ _ _ _ _ _ _ _ _ _ _ _ _ _ _ _ _ _]
          frame 0, Default {
            # "switch to manual\nSet intake speed to slow\nLower intake\nStart intake motor"
            n361 = shared-variable ".\\Shared Variables.lvlib\\Driver.lvlib\\driverButton10"(TRUE ("driverButton10")) -> (error out=w803:errorcluster)  [unwired: 1 in]
            n362 = shared-variable ".\\Shared Variables.lvlib\\Misc..lvlib\\Desired Intake Speed"(0.2 ("Intake RPM"), error in=w803) -> (error out=w802:errorcluster)
            n363 = shared-variable ".\\Shared Variables.lvlib\\Driver.lvlib\\driverButton6"(TRUE ("driverButton6"), error in=w802) -> (error out=w805:errorcluster)
            n364 = shared-variable ".\\Shared Variables.lvlib\\Driver.lvlib\\driverButton1"(TRUE ("driverButton1"), error in=w805) -> (error out=w799:errorcluster)
            n365 = shared-variable ".\\Shared Variables.lvlib\\Driver.lvlib\\driverButton7"(FALSE ("driverButton8"), error in=w799) -> ()  [unwired: 1 out]
          }
          frame 4 {
            # "wait for intake to lower"
            n366 = call "Delay.vi"("Timer Going?"=TRUE, "Time to Wait (ms)"=450.0) -> ("Time Up"=w819:bool)
            n367 = Select(t=7, s=w819, f=w816) -> (s? t:f=w818:i32)
          }
          frame 7 {
            # "turn intake off\nset intake speed to ful"
            n368 = call <vilib>:"WPI_EncoderGet.vi"("EncoderDevRef"=w868) -> ("Distance"=w861:dbl)  [unwired: 5 in, 5 out]
            n369 = call <vilib>:"WPI_EncoderGet.vi"("EncoderDevRef"=w867) -> ("Distance"=w860:dbl)  [unwired: 5 in, 5 out]
            n370 = Add(x=w861, y=w860) -> (x+y=w859:dbl)
            n371 = Divide(x=w859, y=2.0) -> (x/y=w824:dbl)
            n372 = Divide(x=250.0, y=360.0) -> (x/y=w828:dbl)
            n373 = Multiply(x="auto 3 distance 6", y=w828) -> (x*y=w865:dbl)
            n374 = Multiply(x=w828, y="Slowdown Distance") -> (x*y=w849:dbl)
            n375 = Select(t=w849, s=w831, f="Slowdown Distance") -> (s? t:f=w846:dbl)
            n376 = Multiply(x=w828, y="Ball Drop Distance") -> (x*y=w830:dbl)
            n377 = Select(t=w830, s=w831, f="Ball Drop Distance") -> (s? t:f=w827:dbl)
            n378 = Select(t=w865, s=w831, f="auto 3 distance 6") -> (s? t:f=w826:dbl)
            n379 = Subtract(x=w826, y=w846) -> (x-y=w847:dbl)
            n380 = Subtract(x=w826, y=w827) -> (x-y=w825:dbl)
            n381 = Greater?(x=w824, y=w847) -> (0:w833:bool)
            n382 = Greater?(x=w824, y=w825) -> (0:w823:bool)
            n383 = Greater?(x=w824, y=w826) -> (0:w851:bool)
            n384 = disable-structure shown="Disabled" {
              disable-tunnel: w851 -> [w870 _]
              disable-tunnel: [w869 _] -> w850
              frame Disabled {
                # "run intake\ndrive"
                n385 = Select(t=0.0, s=w870, f=-0.8 ("driverJoystickAxis2")) -> (s? t:f=w871:dbl)
                n386 = shared-variable ".\\Shared Variables.lvlib\\Driver.lvlib\\driverJoystickAxis2"(w871) -> (error out=w869:errorcluster)  [unwired: 1 in]
              }
              frame Enabled {
              }
            }
            n387 = Subtract(x=w826, y=w824) -> (x-y=w840:dbl)
            n388 = Divide(x=w840, y=w846) -> (x/y=w845:dbl)
            n389 = Multiply(x=w845, y=-0.3) -> (x*y=w843:dbl)
            n390 = Select(t=w843, s=w833, f=-0.8) -> (s? t:f=w836:dbl)
            n391 = Add(x=w836, y=0.0) -> (x+y=w834:dbl)
            n392 = In Range and Coerce(upper limit=3.0, x=w840, lower limit=-3.0) -> (In Range?=w839:bool)  [unwired: 1 out]
            n393 = Select(t=32, s=w839, f=w857) -> (s? t:f=w866:i32)
            n394 = shared-variable ".\\Shared Variables.lvlib\\Driver.lvlib\\driverButton6"(TRUE ("driverButton6")) -> ()  [unwired: 1 in, 1 out]
            n395 = Not(x=w823) -> ()  [unwired: 1 out]
            n396 = Select(t=0.0, s=w839, f=w834) -> (s? t:f=w837:dbl)
            n397 = shared-variable ".\\Shared Variables.lvlib\\Misc..lvlib\\Desired Intake Speed"(1.0 ("Desired Intake Speed"), error in=w850) -> ()  [unwired: 1 out]
            n398 = shared-variable ".\\Shared Variables.lvlib\\Driver.lvlib\\driverJoystickAxis2"(w837) -> ()  [unwired: 1 in, 1 out]
            n399 = shared-variable ".\\Shared Variables.lvlib\\Driver.lvlib\\driverButton1"(FALSE ("driverButton1")) -> ()  [unwired: 1 in, 1 out]
            n400 = Get Date/Time In Seconds() -> (seconds since 1Jan1904=w821:timestamp)
          }
          frame 3 {
            # "Wait 300ms after stoping"
            n401 = call "Delay.vi"("Timer Going?"=TRUE, "Time to Wait (ms)"=300.0) -> ("Time Up"=w881:bool)
            n402 = Select(t=9 ("x"), s=w881, f=w879) -> (s? t:f=w878:i32)
          }
          frame 9 {
            # "wait for encoder to stop"
            n403 = call <vilib>:"WPI_EncoderGet.vi"("EncoderDevRef"=w892) -> ("Stopped"=w890:bool)  [unwired: 5 in, 5 out]
            n404 = call <vilib>:"WPI_EncoderGet.vi"("EncoderDevRef"=w891) -> ("Stopped"=w889:bool)  [unwired: 5 in, 5 out]
            n405 = And(x=w890, y=w889) -> (x .and. y?=w888:bool)
            n406 = Select(t=32, s=w888, f=w894) -> (s? t:f=w893:i32)
            n407 = shared-variable ".\\Shared Variables.lvlib\\Driver.lvlib\\driverButton6"(FALSE ("driverButton6")) -> ()  [unwired: 1 in, 1 out]
            n408 = Get Date/Time In Seconds() -> (seconds since 1Jan1904=w884:timestamp)
          }
          frame 32 {
            (unwired) FALSE ("driverButton6")
            w919 = 1.0 ("f")
            # "Turn robot X degrees"
            n409 = To Double Precision Float(number=w910) -> (double precision float=w914:dbl)
            n410 = Absolute Value(x=w901) -> (abs(x)=w900:dbl)
            n411 = Get Date/Time In Seconds() -> (seconds since 1Jan1904=w916:timestamp)
            n412 = shared-variable ".\\Shared Variables.lvlib\\Driver.lvlib\\driverJoystickAxis2"(0.0 ("driverJoystickAxis2")) -> ()  [unwired: 1 in, 1 out]
            n413 = To Double Precision Float(number=w916) -> (double precision float=w915:dbl)
            n414 = Add(x=w914, y="Abort Turn 2") -> (x+y=w918:dbl)
            n415 = shared-variable ".\\Shared Variables.lvlib\\Dashboard Variables.lvlib\\Kinect Status"() -> (w909:bool)  [unwired: 1 in, 1 out]
            "Turn Left 3" <- w909
            n416 = Or(x=w909, y=w908) -> (x .or. y?=w907:bool)
            n417 = Less?(x=w918, y=w915) -> (x < y?=w913:bool)
            n418 = Select(t="Left Rotate 2", s=w907, f=0.0) -> (s? t:f=w905:dbl)
            n419 = Negate(x=w919) -> ()  [unwired: 1 out]
            n420 = Select(t="left turn angle 4", s=w907, f="right turn angle 4") -> (s? t:f=w898:dbl)
            n421 = Absolute Value(x=w898) -> (abs(x)=w897:dbl)
            n422 = Divide(x=w897, y=2.0) -> (x/y=w895:dbl)
            n423 = Less?(x=w900, y=w895) -> (x < y?=w899:bool)
            n424 = shared-variable ".\\Shared Variables.lvlib\\Driver.lvlib\\driverButton6"(w899) -> ()  [unwired: 1 in, 1 out]
            n425 = Select(t="Left Strafe 2", s=w907, f=w919) -> (s? t:f=w920:dbl)
            n426 = disable-structure shown="Disabled" {
              frame Disabled {
                n427 = shared-variable ".\\Shared Variables.lvlib\\Driver.lvlib\\driverJoystickAxis1"(0.0 ("driverJoystickAxis1")) -> ()  [unwired: 1 in, 1 out]
              }
              frame Enabled {
              }
            }
            n428 = shared-variable ".\\Shared Variables.lvlib\\Driver.lvlib\\driverJoystickAxis1"(w920) -> ()  [unwired: 1 in, 1 out]
            n429 = Subtract(x=w901, y=w898) -> (x-y=w926:dbl)
            n430 = shared-variable ".\\Shared Variables.lvlib\\Driver.lvlib\\driverJoystickAxis3"(w905) -> ()  [unwired: 1 in, 1 out]
            n431 = Absolute Value(x=w926) -> (abs(x)=w925:dbl)
            n432 = Less Or Equal?(x=w925, y=3.0) -> (x <= y?=w912:bool)
            n433 = Or(x=w912, y=w913) -> (x .or. y?=w911:bool)
            n434 = Select(t=33, s=w911, f=w923) -> (s? t:f=w927:i32)
          }
          frame 33 {
            w931 = 0.0 ("driverJoystickAxis1")
            # "This loop is for settling down after turning the robot.\nIncrease this loop to ensure Ball 1 goes through in \n2nd 5-second period."
            # "Wait for settling after turn"
            n435 = shared-variable ".\\Shared Variables.lvlib\\Driver.lvlib\\driverJoystickAxis1"(0.0 ("driverJoystickAxis1")) -> ()  [unwired: 1 in, 1 out]
            n436 = To Double Precision Float(number=w932) -> (double precision float=w933:dbl)
            n437 = shared-variable ".\\Shared Variables.lvlib\\Driver.lvlib\\driverJoystickAxis3"(w931) -> ()  [unwired: 1 in, 1 out]
            n438 = shared-variable ".\\Shared Variables.lvlib\\Driver.lvlib\\driverJoystickAxis1"(w931) -> ()  [unwired: 1 in, 1 out]
            n439 = while {
              tunnel: w933 -> [w943]
              stop <- w946 continue-if-true
              n440 = Wait (ms)(milliseconds to wait=u32 10) -> ()  [unwired: 1 out]
              n441 = Get Date/Time In Seconds() -> (seconds since 1Jan1904=w949:timestamp)
              n442 = To Double Precision Float(number=w949) -> (double precision float=w947:dbl)
              n443 = Add(x=w943, y="When To Start Firing 3") -> (x+y=w948:dbl)
              n444 = Greater?(x=w948, y=w947) -> (0:w946:bool)
            }
            n445 = shared-variable ".\\Shared Variables.lvlib\\Driver.lvlib\\driverJoystickAxis2"(w931) -> ()  [unwired: 1 in, 1 out]
            n446 = call "Delay.vi"("Timer Going?"=TRUE, "Time to Wait (ms)"=250.0) -> ("Time Up"=w935:bool)
            n447 = Select(t=10, s=w935, f=w938) -> (s? t:f=w941:i32)
          }
          frame 10 {
            # "Combine states 10 & 11"
            # "Fire 1"
            # "fire"
            n448 = Increment(x=w953) -> (x+1=w956:i32)
            n449 = Greater Or Equal?(x=w950, y=w954) -> (x >= y?=w955:bool)
            n450 = shared-variable ".\\Shared Variables.lvlib\\Driver.lvlib\\driverButton8"(TRUE ("driverButton8")) -> ()  [unwired: 1 in, 1 out]
            n451 = Select(t=w956, s=w955, f=w953) -> (s? t:f=w952:i32)
          }
          frame 11 {
            # "wait for fire to comlete"
            n452 = call "Delay.vi"("Timer Going?"=TRUE, "Time to Wait (ms)"=w960) -> ("Time Up"=w967:bool)
            n453 = Select(t=13, s=w967, f=w966) -> (s? t:f=w965:i32)
          }
          frame 13 {
            # "wait for arm to come down"
            n454 = call <vilib>:"WPI_EncoderReset.vi"("EncoderDevRef"=w971) -> ()  [unwired: 9 in, 2 out]
            n455 = call <vilib>:"WPI_AnalogChannelGetVoltage.vi"("AIDeviceRef"=w980) -> ("Voltage"=w979:dbl)  [unwired: 8 in, 2 out]
            n456 = Increment(x=w982) -> (x+1=w983:i32)
            n457 = shared-variable ".\\Shared Variables.lvlib\\Driver.lvlib\\driverButton8"(FALSE ("driverButton8")) -> ()  [unwired: 1 in, 1 out]
            n458 = shared-variable ".\\Shared Variables.lvlib\\Driver.lvlib\\driverButton7"(TRUE ("driverButton8")) -> ()  [unwired: 1 in, 1 out]
            n459 = call <vilib>:"WPI_EncoderReset.vi"("EncoderDevRef"=w970) -> ()  [unwired: 9 in, 2 out]
            n460 = In Range and Coerce(upper limit=5.0, x=w979, lower limit=1.8) -> (In Range?=w976:bool)  [unwired: 1 out]
            n461 = Select(t=w983, s=w976, f=w982) -> (s? t:f=w981:i32)
          }
          frame 14 {
            # "intake ball 2"
            n462 = call <vilib>:"WPI_EncoderGet.vi"("EncoderDevRef"=w999) -> ("Distance"=w1003:dbl)  [unwired: 5 in, 5 out]
            n463 = call <vilib>:"WPI_EncoderGet.vi"("EncoderDevRef"=w1000) -> ("Distance"=w1004:dbl)  [unwired: 5 in, 5 out]
            n464 = Increment(x=w1008) -> (x+1=w1007:i32)
            n465 = Add(x=w1004, y=w1003) -> (x+y=w1002:dbl)
            n466 = shared-variable ".\\Shared Variables.lvlib\\Driver.lvlib\\driverButton7"(FALSE ("driverButton8")) -> (error out=w1013:errorcluster)  [unwired: 1 in]
            n467 = Divide(x=w1002, y=2.0) -> (x/y=w992:dbl)
            n468 = Absolute Value(x=w992) -> (abs(x)=w991:dbl)
            n469 = Divide(x=250.0, y=360.0) -> (x/y=w988:dbl)
            n470 = shared-variable ".\\Shared Variables.lvlib\\Driver.lvlib\\driverButton6"(TRUE ("driverButton1"), error in=w1013) -> (error out=w1009:errorcluster)
            n471 = Multiply(x="BackupLimit 2", y=w988) -> (x*y=w990:dbl)
            n472 = Select(t=w990, s=w986, f="BackupLimit 2") -> (s? t:f=w984:dbl)
            n473 = Greater Or Equal?(x=w991, y=w984) -> (x >= y?=w998:bool)
            n474 = Or(x=w998, y=w1005) -> (x .or. y?=w997:bool)
            n475 = Select(t=w1007, s=w997, f=w1008) -> (s? t:f=w1006:i32)
            n476 = Select(t=0.0, s=w997, f="BackupSpeed 2") -> (s? t:f=w994:dbl)
            n477 = shared-variable ".\\Shared Variables.lvlib\\Driver.lvlib\\driverJoystickAxis2"(w994) -> ()  [unwired: 1 in, 1 out]
            n478 = shared-variable ".\\Shared Variables.lvlib\\Misc..lvlib\\Desired Intake Speed"(1.0 ("Desired Intake Speed"), error in=w1009) -> ()  [unwired: 1 out]
          }
          frame 15 {
            # "Consider decreasing settling time"
            # "wait for intake to finish"
            n479 = call <vilib>:"WPI_AnalogChannelGetVoltage.vi"("AIDeviceRef"=w1018) -> ("Voltage"=w1017:dbl)  [unwired: 8 in, 2 out]
            n480 = In Range and Coerce(upper limit=5.0, x=w1017, lower limit=0.6) -> (In Range?=w1026:bool)  [unwired: 1 out]
            n481 = call "Stable.vi"("Eval Period (sec)"=0.03, "Signal Input"=w1026) -> ("Stable"=w1024:bool)  [unwired: 9 in]
            n482 = Increment(x=w1023) -> (x+1=w1022:i32)
            n483 = Select(t=w1022, s=w1024, f=w1023) -> (s? t:f=w1021:i32)
          }
          frame 16 {
            # "raise intake\nstop intaking"
            n484 = shared-variable ".\\Shared Variables.lvlib\\Driver.lvlib\\driverButton6"(FALSE ("driverButton1")) -> (error out=w1032:errorcluster)  [unwired: 1 in]
            n485 = shared-variable ".\\Shared Variables.lvlib\\Driver.lvlib\\driverButton1"(TRUE ("driverButton1"), error in=w1032) -> ()  [unwired: 1 out]
            n486 = Increment(x=w1035) -> (x+1=w1034:i32)
          }
          frame 17 {
            # "wait for intake to raise\nDelay for CMD"
            n487 = call "Delay.vi"("Timer Going?"=TRUE, "Time to Wait (ms)"=100.0) -> ("Time Up"=w1044:bool)
            n488 = Select(t=27, s=w1044, f=w1042) -> (s? t:f=w1041:i32)
          }
          frame 27 {
            # "wait for intake to raise\nDelay for CMD"
            n489 = shared-variable ".\\Shared Variables.lvlib\\Driver.lvlib\\driverButton1"(FALSE ("driverButton1")) -> (error out=w1047:errorcluster)  [unwired: 1 in]
            n490 = shared-variable ".\\Shared Variables.lvlib\\Misc..lvlib\\Desired Intake Speed"(0.2 ("Desired Intake Speed"), error in=w1047) -> ()  [unwired: 1 out]
            n491 = call "Delay.vi"("Timer Going?"=TRUE, "Time to Wait (ms)"=100.0) -> ("Time Up"=w1056:bool)
            n492 = Select(t=28, s=w1056, f=w1054) -> (s? t:f=w1053:i32)
          }
          frame 28 {
            # "Typically 250ms"
            # "wait for intake to raise\nDelay for CMD"
            n493 = shared-variable ".\\Shared Variables.lvlib\\Driver.lvlib\\driverButton6"(TRUE ("driverButton1")) -> ()  [unwired: 1 in, 1 out]
            n494 = call "Delay.vi"("Timer Going?"=TRUE, "Time to Wait (ms)"=500.0) -> ("Time Up"=w1066:bool)
            n495 = Select(t=20, s=w1066, f=w1064) -> (s? t:f=w1063:i32)
          }
          frame 20 {
            # "run intake motor\n lower intake"
            n496 = Increment(x=w1073) -> (x+1=w1072:i32)
            n497 = shared-variable ".\\Shared Variables.lvlib\\Driver.lvlib\\driverButton1"(TRUE ("driverButton1")) -> ()  [unwired: 1 in, 1 out]
          }
          frame 21 {
            # "Consider decreasing settling time"
            # "wait for intake to lower\n(450ms)"
            n498 = Increment(x=w1078) -> (x+1=w1081:i32)
            n499 = call "Delay.vi"("Timer Going?"=TRUE, "Time to Wait (ms)"=450.0 ("Wait for Intake to Lower (450ms)")) -> ("Time Up"=w1080:bool)
            n500 = Select(t=w1081, s=w1080, f=w1078) -> (s? t:f=w1077:i32)
          }
          frame 22 {
            # "stop running intake motor\nfire\nDe-Assert Lower Intake"
            n501 = Increment(x=w1087) -> (x+1=w1088:i32)
            n502 = Greater Or Equal?(x=w1083, y=w1086) -> (x >= y?=w1085:bool)
            n503 = Select(t=w1088, s=w1085, f=w1087) -> (s? t:f=w1089:i32)
            n504 = shared-variable ".\\Shared Variables.lvlib\\Driver.lvlib\\driverButton1"(FALSE ("driverButton1")) -> (error out=w1092:errorcluster)  [unwired: 1 in]
            n505 = shared-variable ".\\Shared Variables.lvlib\\Driver.lvlib\\driverButton6"(FALSE ("driverButton1"), error in=w1092) -> (error out=w1094:errorcluster)
            n506 = shared-variable ".\\Shared Variables.lvlib\\Driver.lvlib\\driverButton8"(TRUE ("driverButton1"), error in=w1094) -> ()  [unwired: 1 out]
          }
          frame 23 {
            # "wait for fire"
            n507 = Increment(x=w1102) -> (x+1=w1105:i32)
            n508 = call "Delay.vi"("Timer Going?"=TRUE, "Time to Wait (ms)"=w1097) -> ("Time Up"=w1104:bool)
            n509 = Select(t=w1105, s=w1104, f=w1102) -> (s? t:f=w1101:i32)
          }
          frame 24 {
            # "stop fire\nretract arm"
            n510 = shared-variable ".\\Shared Variables.lvlib\\Driver.lvlib\\driverButton8"(FALSE ("driverButton8")) -> (error out=w1109:errorcluster)  [unwired: 1 in]
            n511 = shared-variable ".\\Shared Variables.lvlib\\Driver.lvlib\\driverButton7"(TRUE ("driverButton8"), error in=w1109) -> ()  [unwired: 1 out]
            n512 = Increment(x=w1111) -> (x+1=w1110:i32)
          }
          frame 25 {
            # "wait for retract"
            n513 = call <vilib>:"WPI_AnalogChannelGetVoltage.vi"("AIDeviceRef"=w1117) -> ("Voltage"=w1121:dbl)  [unwired: 8 in, 2 out]
            n514 = In Range and Coerce(upper limit=5.0, x=w1121, lower limit=1.5) -> (In Range?=w1118:bool)  [unwired: 1 out]
            n515 = Increment(x=w1122) -> (x+1=w1124:i32)
            n516 = Select(t=w1124, s=w1118, f=w1122) -> (s? t:f=w1123:i32)
          }
          frame 26 {
            # "wait for fire"
            # "bring intake arm up\nEND AUTO"
            n517 = shared-variable ".\\Shared Variables.lvlib\\Driver.lvlib\\driverButton7"(FALSE ("driverButton8")) -> (error out=w1134:errorcluster)  [unwired: 1 in]
            n518 = shared-variable ".\\Shared Variables.lvlib\\Driver.lvlib\\driverButton1"(TRUE ("driverButton1"), error in=w1134) -> ()  [unwired: 1 out]
            n519 = call "Delay.vi"("Timer Going?"=TRUE, "Time to Wait (ms)"=50.0) -> ("Time Up"=w1128:bool)
            n520 = Select(t=29, s=w1128, f=w1126) -> (s? t:f=w1125:i32)
          }
          frame 29 {
            w1140 = 0.0 ("Desired Intake Speed")
            n521 = shared-variable ".\\Shared Variables.lvlib\\Driver.lvlib\\driverButton1"(FALSE ("driverButton1")) -> ()  [unwired: 1 in, 1 out]
            n522 = shared-variable ".\\Shared Variables.lvlib\\Misc..lvlib\\Desired Intake Speed"(w1140) -> (error out=w1139:errorcluster)  [unwired: 1 in]
            n523 = shared-variable ".\\Shared Variables.lvlib\\Driver.lvlib\\driverJoystickAxis3"(w1140, error in=w1139) -> (error out=w1138:errorcluster)
            n524 = shared-variable ".\\Shared Variables.lvlib\\Driver.lvlib\\driverJoystickAxis1"(w1140, error in=w1138) -> (error out=w1137:errorcluster)
            n525 = shared-variable ".\\Shared Variables.lvlib\\Driver.lvlib\\driverJoystickAxis2"(w1140, error in=w1137) -> ()  [unwired: 1 out]
          }
        }
        n526 = Select(t=cluster{"output high":dbl, "output low":dbl} {"output high"=0.0, "output low"=0.0} ("output range"), s=w784, f=cluster{"output high":dbl, "output low":dbl} {"output high"=0.6, "output low"=-0.6} ("output range")) -> (s? t:f=w785:cluster{"output high":dbl, "output low":dbl})
        n527 = call-poly <vilib>:"PID.vi"("reinitialize? (F)"=w784, "output range"=w785, "PID gains"=w791, "process variable"=w783, "setpoint"=w792) -> ("output"=w794:dbl)  [unwired: 5 in, 1 out]
        n528 = shared-variable ".\\Shared Variables.lvlib\\Driver.lvlib\\driverJoystickAxis3"(w794) -> ()  [unwired: 1 in, 1 out]
        "State 4" <- w793
      }
    }
    frame 64 {
      n529 = call <vilib>:"WPI_EncoderRefNum Registry Get.vi"("refnum name"="leftWheelEncoder") -> ("EncoderDevRef"=w1167:T3)  [unwired: 9 in, 1 out]
      n530 = call <vilib>:"WPI_EncoderRefNum Registry Get.vi"("refnum name"="rightWheelEncoder") -> ("EncoderDevRef"=w1166:T3)  [unwired: 9 in, 1 out]
      n531 = call <vilib>:"WPI_GyroRefNum Registry Get.vi"("refnum name"="yawGyro") -> ("error out"=w1154:errorcluster, "GyroDevRef"=w1155:T7)  [unwired: 9 in]
      n532 = call <vilib>:"WPI_GyroReset.vi"("error in (no error)"=w1154, "GyroDevRef"=w1155) -> ("GyroDevRef"=w1152:T7)  [unwired: 8 in, 1 out]
      n533 = call <vilib>:"WPI_EncoderReset.vi"("EncoderDevRef"=w1167) -> ("EncoderDevRef"=w1162:T3)  [unwired: 9 in, 1 out]
      n534 = call <vilib>:"WPI_EncoderReset.vi"("EncoderDevRef"=w1166) -> ("EncoderDevRef"=w1161:T3)  [unwired: 9 in, 1 out]
      n535 = call <vilib>:"WPI_AnalogChannelRefNum Registry Get.vi"("refnum name"="irProximDistCatapult") -> ("AIDeviceRef"=w1160:T10)  [unwired: 9 in, 1 out]
      n536 = call <vilib>:"WPI_AnalogChannelRefNum Registry Get.vi"("refnum name"="irProximDistCatDown") -> ("AIDeviceRef"=w1156:T10)  [unwired: 9 in, 1 out]
      n537 = Get Date/Time In Seconds() -> (seconds since 1Jan1904=w1148:timestamp)
      n538 = call <vilib>:"WPI_DigitalInputRefNum Registry Get.vi"("refnum name"="irProximSwitchLeftIntake") -> ("DigitalInputDevRef"=w1149:T11)  [unwired: 9 in, 1 out]
      n539 = while {
        tunnel: w1163 -> [w1202]
        tunnel: w1162 -> [w1201]
        tunnel: w1161 -> [w1200]
        tunnel: w1160 -> [w1176]
        shift-right: [w1194] -> _
        shift-left: 0 -> [w1197]
        tunnel: w1156 -> [w1175]
        tunnel: w1152 -> [_]
        tunnel: w1151 -> [w1195]
        tunnel: w1148 -> [w1192]
        tunnel: w1149 -> [w1184]
        shift-right: [w1174] -> _
        shift-left: w1148 -> [w1173]
        tunnel: w1147 -> [w1171]
        tunnel: w1146 -> [w1170]
        stop <- FALSE stop-if-true
        n540 = shared-variable ".\\Shared Variables.lvlib\\Sensors-Actuators.lvlib\\Gyro.lvlib\\yawGyro"() -> (w1187:dbl)  [unwired: 1 in, 1 out]
        "Waveform Chart 4" <- w1187
        n541 = call <vilib>:"WPI_DigitalInputGetValue.vi"("DigitalInputDevRef"=w1184) -> ("Value"=w1185:bool)  [unwired: 8 in, 2 out]
        n542 = Wait (ms)(milliseconds to wait=u32 25) -> ()  [unwired: 1 out]
        n543 = call <vilib>:"WPI_AnalogChannelGetVoltage.vi"("AIDeviceRef"=w1175) -> ("Voltage"=w1177:dbl)  [unwired: 8 in, 2 out]
        n544 = Not(x=w1185) -> (.not. x?=w1183:bool)
        n545 = call-poly <vilib>:"PID Control Input Filter.vi"("input"=w1177) -> ("output"=w1186:dbl)  [unwired: 4 in]
        n546 = Boolean To (0,1)(Boolean=w1183) -> (0, 1=w1179:i16)
        n547 = call-poly <vilib>:"PID Control Input Filter.vi"("input"=w1179) -> ("output"=w1182:dbl)  [unwired: 4 in]
        n548 = call <userlib>:"Schmitt Trigger.vi"("lo"=sgl 0.1 ("High to Low\nTransition"), "in"=w1182, "hi"=sgl 0.9 ("Low to High\nTransition")) -> ("out"=w1178:bool)  [unwired: 1 out]
        n549 = shared-variable ".\\Shared Variables.lvlib\\Quick Change Params.lvlib\\FireDelay"() -> (w1169:dbl)  [unwired: 1 in, 1 out]
        n550 = case shown="13" w1197 {
          selector: w1197 -> [_ w1220 w1262 w1283 w1298 w1329 w1343 w1358 w1371 w1387 w1413 w1428 w1440 w1447 w1459 w1469 w1478 w1483 w1492 w1507 w1516 w1527 w1531 w1551]
          tunnel: [4 ("t") w1222 w1270 w1282 w1297 w1333 w1346 w1357 w1370 w1386 w1411 w1426 w1439 w1446 w1458 w1468 w1477 w1482 w1494 w1506 w1515 w1528 w1530 w1551] -> w1194
          tunnel: w1202 -> [_ _ w1236 _ _ _ _ _ _ _ w1391 _ _ _ _ _ _ _ _ _ _ _ _ _]
          tunnel: w1201 -> [_ _ w1272 _ w1296 _ _ _ _ w1375 w1405 _ _ _ _ _ _ _ _ _ _ _ _ _]
          tunnel: w1200 -> [_ _ w1271 _ w1295 _ _ _ _ w1376 w1404 _ _ _ _ _ _ _ _ _ _ _ _ _]
          tunnel: w1175 -> [_ _ _ _ _ _ _ _ _ w1385 _ _ _ _ _ _ _ _ _ _ _ w1522 _ _]
          tunnel: [0.0 ("setpoint") 0.0 ("setpoint") 0.0 ("setpoint") 0.0 ("setpoint") 0.0 ("setpoint") w1309 w1345 w1363 w1369 w1380 w1417 w1425 w1436 w1445 w1457 w1467 w1476 w1481 w1496 w1505 w1513 w1521 w1538 w1550] -> w1196
          tunnel: w1187 -> [_ _ _ _ _ w1311 w1345 w1363 w1369 w1380 w1417 w1425 w1436 w1445 w1457 w1467 w1476 w1481 w1496 w1505 w1513 w1521 w1538 w1550]
          tunnel: [FALSE FALSE FALSE FALSE FALSE FALSE TRUE TRUE TRUE TRUE TRUE TRUE TRUE TRUE TRUE TRUE TRUE TRUE TRUE TRUE TRUE TRUE TRUE TRUE] -> w1188
          tunnel: w1192 -> [w1205 w1216 _ w1278 _ _ w1337 w1356 w1366 w1374 w1398 w1421 w1434 w1442 w1451 w1463 w1473 w1479 w1489 w1503 w1511 w1519 w1536 w1548]
          tunnel: w1186 -> [_ _ _ _ _ _ _ w1359 _ _ _ _ _ _ _ _ _ _ w1491 _ _ _ _ _]
          tunnel: w1178 -> [_ _ _ _ _ _ _ _ _ _ w1410 _ _ _ _ _ _ _ _ _ _ _ _ _]
          tunnel: w1176 -> [_ _ _ _ _ _ _ _ _ _ _ w1423 _ _ _ _ _ _ _ _ _ _ _ _]
          tunnel: [w1205 w1216 w1226 w1278 w1288 w1317 w1337 w1356 w1366 w1374 w1398 w1421 w1434 w1442 w1451 w1463 w1473 w1479 w1489 w1503 w1511 w1519 w1536 w1548] -> w1174
          tunnel: w1173 -> [_ _ _ _ _ w1317 _ _ _ _ _ _ _ _ _ _ _ _ _ _ _ _ _ _]
          tunnel: "Catapult Down 3" -> [_ _ _ _ _ _ _ w1355 _ _ _ _ _ _ _ _ _ _ w1488 _ _ _ _ _]
          tunnel: w1169 -> [_ _ _ _ _ _ _ _ w1365 _ _ _ _ _ _ _ _ _ _ w1502 _ _ _ _]
          tunnel: w1171 -> [_ _ _ _ _ w1315 _ _ _ _ _ _ _ _ _ _ _ _ _ _ _ _ _ _]
          tunnel: w1170 -> [_ _ _ _ _ _ _ _ _ _ _ _ _ _ _ _ _ _ _ _ _ _ _ _]
          frame 0, Default {
            # "switch to manual\nSet intake speed to slow\nLower intake\nStart intake motor"
            n551 = shared-variable ".\\Shared Variables.lvlib\\Driver.lvlib\\driverButton10"(TRUE ("driverButton10")) -> (error out=w1207:errorcluster)  [unwired: 1 in]
            n552 = shared-variable ".\\Shared Variables.lvlib\\Misc..lvlib\\Desired Intake Speed"(0.2 ("Intake RPM"), error in=w1207) -> (error out=w1206:errorcluster)
            n553 = shared-variable ".\\Shared Variables.lvlib\\Driver.lvlib\\driverButton6"(TRUE ("driverButton6"), error in=w1206) -> (error out=w1209:errorcluster)
            n554 = shared-variable ".\\Shared Variables.lvlib\\Driver.lvlib\\driverButton1"(TRUE ("driverButton1"), error in=w1209) -> (error out=w1203:errorcluster)
            n555 = shared-variable ".\\Shared Variables.lvlib\\Driver.lvlib\\driverButton7"(FALSE ("driverButton8"), error in=w1203) -> ()  [unwired: 1 out]
          }
          frame 4 {
            # "wait for intake to lower"
            n556 = call "Delay.vi"("Timer Going?"=TRUE, "Time to Wait (ms)"=450.0) -> ("Time Up"=w1223:bool)
            n557 = Select(t=7, s=w1223, f=w1220) -> (s? t:f=w1222:i32)
          }
          frame 7 {
            # "turn intake off\nset intake speed to ful"
            n558 = call <vilib>:"WPI_EncoderGet.vi"("EncoderDevRef"=w1272) -> ("Distance"=w1266:dbl)  [unwired: 5 in, 5 out]
            n559 = call <vilib>:"WPI_EncoderGet.vi"("EncoderDevRef"=w1271) -> ("Distance"=w1265:dbl)  [unwired: 5 in, 5 out]
            n560 = Add(x=w1266, y=w1265) -> (x+y=w1264:dbl)
            n561 = shared-variable ".\\Shared Variables.lvlib\\Quick Change Params.lvlib\\AutoDistance"() -> (w1225:dbl)  [unwired: 1 in, 1 out]
            n562 = Divide(x=w1264, y=2.0) -> (x/y=w1229:dbl)
            n563 = Divide(x=250.0, y=360.0) -> (x/y=w1233:dbl)
            n564 = Multiply(x=w1225, y=w1233) -> (x*y=w1269:dbl)
            n565 = Multiply(x=w1233, y="Slowdown Distance 2") -> (x*y=w1254:dbl)
            n566 = Select(t=w1254, s=w1236, f="Slowdown Distance 2") -> (s? t:f=w1251:dbl)
            n567 = Multiply(x=w1233, y="Ball Drop Distance 2") -> (x*y=w1235:dbl)
            n568 = Select(t=w1235, s=w1236, f="Ball Drop Distance 2") -> (s? t:f=w1232:dbl)
            n569 = Select(t=w1269, s=w1236, f=w1225) -> (s? t:f=w1231:dbl)
            n570 = Subtract(x=w1231, y=w1251) -> (x-y=w1252:dbl)
            n571 = Subtract(x=w1231, y=w1232) -> (x-y=w1230:dbl)
            n572 = Greater?(x=w1229, y=w1252) -> (0:w1238:bool)
            n573 = Greater?(x=w1229, y=w1230) -> (0:w1228:bool)
            n574 = Greater?(x=w1229, y=w1231) -> (0:w1256:bool)
            n575 = disable-structure shown="Disabled" {
              disable-tunnel: w1256 -> [w1274 _]
              disable-tunnel: [w1273 _] -> w1255
              frame Disabled {
                # "run intake\ndrive"
                n576 = Select(t=0.0, s=w1274, f=-0.8 ("driverJoystickAxis2")) -> (s? t:f=w1275:dbl)
                n577 = shared-variable ".\\Shared Variables.lvlib\\Driver.lvlib\\driverJoystickAxis2"(w1275) -> (error out=w1273:errorcluster)  [unwired: 1 in]
              }
              frame Enabled {
              }
            }
            n578 = Subtract(x=w1231, y=w1229) -> (x-y=w1245:dbl)
            n579 = Divide(x=w1245, y=w1251) -> (x/y=w1250:dbl)
            n580 = Multiply(x=w1250, y=-0.3) -> (x*y=w1248:dbl)
            n581 = Select(t=w1248, s=w1238, f=-0.8) -> (s? t:f=w1241:dbl)
            n582 = Add(x=w1241, y=0.0) -> (x+y=w1239:dbl)
            n583 = In Range and Coerce(upper limit=3.0, x=w1245, lower limit=-3.0) -> (In Range?=w1244:bool)  [unwired: 1 out]
            n584 = Select(t=32, s=w1244, f=w1262) -> (s? t:f=w1270:i32)
            n585 = shared-variable ".\\Shared Variables.lvlib\\Driver.lvlib\\driverButton6"(TRUE ("driverButton6")) -> ()  [unwired: 1 in, 1 out]
            n586 = Not(x=w1228) -> ()  [unwired: 1 out]
            n587 = Select(t=0.0, s=w1244, f=w1239) -> (s? t:f=w1242:dbl)
            n588 = shared-variable ".\\Shared Variables.lvlib\\Misc..lvlib\\Desired Intake Speed"(1.0 ("Desired Intake Speed"), error in=w1255) -> ()  [unwired: 1 out]
            n589 = shared-variable ".\\Shared Variables.lvlib\\Driver.lvlib\\driverJoystickAxis2"(w1242) -> ()  [unwired: 1 in, 1 out]
            n590 = shared-variable ".\\Shared Variables.lvlib\\Driver.lvlib\\driverButton1"(FALSE ("driverButton1")) -> ()  [unwired: 1 in, 1 out]
            n591 = Get Date/Time In Seconds() -> (seconds since 1Jan1904=w1226:timestamp)
          }
          frame 3 {
            # "Wait 300ms after stoping"
            n592 = call "Delay.vi"("Timer Going?"=TRUE, "Time to Wait (ms)"=300.0) -> ("Time Up"=w1285:bool)
            n593 = Select(t=9 ("x"), s=w1285, f=w1283) -> (s? t:f=w1282:i32)
          }
          frame 9 {
            # "wait for encoder to stop"
            n594 = call <vilib>:"WPI_EncoderGet.vi"("EncoderDevRef"=w1296) -> ("Stopped"=w1294:bool)  [unwired: 5 in, 5 out]
            n595 = call <vilib>:"WPI_EncoderGet.vi"("EncoderDevRef"=w1295) -> ("Stopped"=w1293:bool)  [unwired: 5 in, 5 out]
            n596 = And(x=w1294, y=w1293) -> (x .and. y?=w1292:bool)
            n597 = Select(t=32, s=w1292, f=w1298) -> (s? t:f=w1297:i32)
            n598 = shared-variable ".\\Shared Variables.lvlib\\Driver.lvlib\\driverButton6"(FALSE ("driverButton6")) -> ()  [unwired: 1 in, 1 out]
            n599 = Get Date/Time In Seconds() -> (seconds since 1Jan1904=w1288:timestamp)
          }
          frame 32 {
            # "When Btn6 Gets turned off\nIs decided by how inflated the ball is.\nHigher inflation, later turn off.\nLower infaltion, earlier turn off."
            # "Turn robot X degrees"
            n600 = To Double Precision Float(number=w1317) -> (double precision float=w1321:dbl)
            n601 = Absolute Value(x=w1311) -> (abs(x)=w1310:dbl)
            n602 = Get Date/Time In Seconds() -> (seconds since 1Jan1904=w1323:timestamp)
            n603 = shared-variable ".\\Shared Variables.lvlib\\Driver.lvlib\\driverButton6"(TRUE ("driverButton6")) -> ()  [unwired: 1 in, 1 out]
            n604 = shared-variable ".\\Shared Variables.lvlib\\Driver.lvlib\\driverJoystickAxis2"(0.0 ("driverJoystickAxis2")) -> ()  [unwired: 1 in, 1 out]
            n605 = shared-variable ".\\Shared Variables.lvlib\\Quick Change Params.lvlib\\RTAngle"() -> (w1302:dbl)  [unwired: 1 in, 1 out]
            n606 = shared-variable ".\\Shared Variables.lvlib\\Quick Change Params.lvlib\\RotatePWR"() -> (w1300:dbl)  [unwired: 1 in, 1 out]
            n607 = shared-variable ".\\Shared Variables.lvlib\\Quick Change Params.lvlib\\LTAngle"() -> (w1301:dbl)  [unwired: 1 in, 1 out]
            n608 = To Double Precision Float(number=w1323) -> (double precision float=w1322:dbl)
            n609 = Add(x=w1321, y="Abort Turn 3") -> (x+y=w1325:dbl)
            n610 = shared-variable ".\\Shared Variables.lvlib\\Quick Change Params.lvlib\\StrafePWR"() -> (w1299:dbl)  [unwired: 1 in, 1 out]
            n611 = shared-variable ".\\Shared Variables.lvlib\\Dashboard Variables.lvlib\\Kinect Status"() -> (w1316:bool)  [unwired: 1 in, 1 out]
            "Turn Left 4" <- w1316
            n612 = Or(x=w1316, y=w1315) -> (x .or. y?=w1314:bool)
            n613 = Less?(x=w1325, y=w1322) -> (x < y?=w1320:bool)
            n614 = Negate(x=w1300) -> (-x=w1304:dbl)
            n615 = Select(t=w1300, s=w1314, f=w1304) -> (s? t:f=w1313:dbl)
            n616 = Negate(x=w1299) -> (-x=w1305:dbl)
            n617 = Select(t=w1301, s=w1314, f=w1302) -> (s? t:f=w1309:dbl)
            n618 = Absolute Value(x=w1309) -> (abs(x)=w1308:dbl)
            n619 = Divide(x=w1308, y=2.0) -> (x/y=w1306:dbl)
            n620 = Less?(x=w1310, y=w1306) -> ()  [unwired: 1 out]
            n621 = Select(t=w1299, s=w1314, f=w1305) -> (s? t:f=w1326:dbl)
            n622 = disable-structure shown="Disabled" {
              frame Disabled {
                n623 = shared-variable ".\\Shared Variables.lvlib\\Driver.lvlib\\driverJoystickAxis1"(0.0 ("driverJoystickAxis1")) -> ()  [unwired: 1 in, 1 out]
              }
              frame Enabled {
              }
            }
            n624 = shared-variable ".\\Shared Variables.lvlib\\Driver.lvlib\\driverJoystickAxis1"(w1326) -> ()  [unwired: 1 in, 1 out]
            n625 = Subtract(x=w1311, y=w1309) -> (x-y=w1332:dbl)
            n626 = shared-variable ".\\Shared Variables.lvlib\\Driver.lvlib\\driverJoystickAxis3"(w1313) -> ()  [unwired: 1 in, 1 out]
            n627 = Absolute Value(x=w1332) -> (abs(x)=w1331:dbl)
            n628 = Less Or Equal?(x=w1331, y=3.0) -> (x <= y?=w1319:bool)
            n629 = Or(x=w1319, y=w1320) -> (x .or. y?=w1318:bool)
            n630 = Select(t=33, s=w1318, f=w1329) -> (s? t:f=w1333:i32)
          }
          frame 33 {
            w1336 = 0.0 ("driverJoystickAxis1")
            # "This loop is for settling down after turning the robot.\nIncrease this loop to ensure Ball 1 goes through in \n2nd 5-second period."
            # "Wait for settling after turn"
            n631 = shared-variable ".\\Shared Variables.lvlib\\Driver.lvlib\\driverJoystickAxis1"(0.0 ("driverJoystickAxis1")) -> ()  [unwired: 1 in, 1 out]
            n632 = shared-variable ".\\Shared Variables.lvlib\\Driver.lvlib\\driverButton6"(FALSE ("driverButton6")) -> ()  [unwired: 1 in, 1 out]
            n633 = To Double Precision Float(number=w1337) -> (double precision float=w1338:dbl)
            n634 = shared-variable ".\\Shared Variables.lvlib\\Driver.lvlib\\driverJoystickAxis3"(w1336) -> ()  [unwired: 1 in, 1 out]
            n635 = shared-variable ".\\Shared Variables.lvlib\\Driver.lvlib\\driverJoystickAxis1"(w1336) -> ()  [unwired: 1 in, 1 out]
            n636 = while {
              tunnel: w1338 -> [w1349]
              stop <- w1351 continue-if-true
              n637 = shared-variable ".\\Shared Variables.lvlib\\Quick Change Params.lvlib\\StartFiringTime"() -> (w1348:dbl)  [unwired: 1 in, 1 out]
              n638 = Wait (ms)(milliseconds to wait=u32 10) -> ()  [unwired: 1 out]
              n639 = Get Date/Time In Seconds() -> (seconds since 1Jan1904=w1354:timestamp)
              n640 = To Double Precision Float(number=w1354) -> (double precision float=w1352:dbl)
              n641 = Add(x=w1349, y=w1348) -> (x+y=w1353:dbl)
              n642 = Greater?(x=w1353, y=w1352) -> (0:w1351:bool)
            }
            n643 = shared-variable ".\\Shared Variables.lvlib\\Driver.lvlib\\driverJoystickAxis2"(w1336) -> ()  [unwired: 1 in, 1 out]
            n644 = call "Delay.vi"("Timer Going?"=TRUE, "Time to Wait (ms)"=250.0) -> ("Time Up"=w1340:bool)
            n645 = Select(t=10, s=w1340, f=w1343) -> (s? t:f=w1346:i32)
          }
          frame 10 {
            # "Combine states 10 & 11"
            # "Fire 1"
            # "fire"
            n646 = Increment(x=w1358) -> (x+1=w1361:i32)
            n647 = Greater Or Equal?(x=w1355, y=w1359) -> (x >= y?=w1360:bool)
            n648 = shared-variable ".\\Shared Variables.lvlib\\Driver.lvlib\\driverButton8"(TRUE ("driverButton8")) -> ()  [unwired: 1 in, 1 out]
            n649 = Select(t=w1361, s=w1360, f=w1358) -> (s? t:f=w1357:i32)
          }
          frame 11 {
            # "wait for fire to comlete"
            n650 = call "Delay.vi"("Timer Going?"=TRUE, "Time to Wait (ms)"=w1365) -> ("Time Up"=w1372:bool)
            n651 = Select(t=13, s=w1372, f=w1371) -> (s? t:f=w1370:i32)
          }
          frame 13 {
            # "wait for arm to come down"
            n652 = call <vilib>:"WPI_EncoderReset.vi"("EncoderDevRef"=w1376) -> ()  [unwired: 9 in, 2 out]
            n653 = call <vilib>:"WPI_AnalogChannelGetVoltage.vi"("AIDeviceRef"=w1385) -> ("Voltage"=w1384:dbl)  [unwired: 8 in, 2 out]
            n654 = Increment(x=w1387) -> (x+1=w1388:i32)
            n655 = shared-variable ".\\Shared Variables.lvlib\\Driver.lvlib\\driverButton8"(FALSE ("driverButton8")) -> ()  [unwired: 1 in, 1 out]
            n656 = shared-variable ".\\Shared Variables.lvlib\\Driver.lvlib\\driverButton7"(TRUE ("driverButton8")) -> ()  [unwired: 1 in, 1 out]
            n657 = call <vilib>:"WPI_EncoderReset.vi"("EncoderDevRef"=w1375) -> ()  [unwired: 9 in, 2 out]
            n658 = In Range and Coerce(upper limit=5.0, x=w1384, lower limit=1.8) -> (In Range?=w1381:bool)  [unwired: 1 out]
            n659 = Select(t=w1388, s=w1381, f=w1387) -> (s? t:f=w1386:i32)
          }
          frame 14 {
            # "intake ball 2"
            n660 = call <vilib>:"WPI_EncoderGet.vi"("EncoderDevRef"=w1404) -> ("Distance"=w1408:dbl)  [unwired: 5 in, 5 out]
            n661 = call <vilib>:"WPI_EncoderGet.vi"("EncoderDevRef"=w1405) -> ("Distance"=w1409:dbl)  [unwired: 5 in, 5 out]
            n662 = Increment(x=w1413) -> (x+1=w1412:i32)
            n663 = Add(x=w1409, y=w1408) -> (x+y=w1407:dbl)
            n664 = shared-variable ".\\Shared Variables.lvlib\\Driver.lvlib\\driverButton7"(FALSE ("driverButton8")) -> (error out=w1418:errorcluster)  [unwired: 1 in]
            n665 = Divide(x=w1407, y=2.0) -> (x/y=w1397:dbl)
            n666 = Absolute Value(x=w1397) -> (abs(x)=w1396:dbl)
            n667 = Divide(x=250.0, y=360.0) -> (x/y=w1393:dbl)
            n668 = shared-variable ".\\Shared Variables.lvlib\\Driver.lvlib\\driverButton6"(TRUE ("driverButton1"), error in=w1418) -> (error out=w1414:errorcluster)
            n669 = Multiply(x="BackupLimit 3", y=w1393) -> (x*y=w1395:dbl)
            n670 = Select(t=w1395, s=w1391, f="BackupLimit 3") -> (s? t:f=w1389:dbl)
            n671 = Greater Or Equal?(x=w1396, y=w1389) -> (x >= y?=w1403:bool)
            n672 = Or(x=w1403, y=w1410) -> (x .or. y?=w1402:bool)
            n673 = Select(t=w1412, s=w1402, f=w1413) -> (s? t:f=w1411:i32)
            n674 = Select(t=0.0, s=w1402, f="BackupSpeed 3") -> (s? t:f=w1399:dbl)
            n675 = shared-variable ".\\Shared Variables.lvlib\\Driver.lvlib\\driverJoystickAxis2"(w1399) -> ()  [unwired: 1 in, 1 out]
            n676 = shared-variable ".\\Shared Variables.lvlib\\Misc..lvlib\\Desired Intake Speed"(1.0 ("Desired Intake Speed"), error in=w1414) -> ()  [unwired: 1 out]
          }
          frame 15 {
            # "Consider decreasing settling time"
            # "wait for intake to finish"
            n677 = call <vilib>:"WPI_AnalogChannelGetVoltage.vi"("AIDeviceRef"=w1423) -> ("Voltage"=w1422:dbl)  [unwired: 8 in, 2 out]
            n678 = In Range and Coerce(upper limit=5.0, x=w1422, lower limit=0.6) -> (In Range?=w1431:bool)  [unwired: 1 out]
            n679 = call "Stable.vi"("Eval Period (sec)"=0.03, "Signal Input"=w1431) -> ("Stable"=w1429:bool)  [unwired: 9 in]
            n680 = Increment(x=w1428) -> (x+1=w1427:i32)
            n681 = Select(t=w1427, s=w1429, f=w1428) -> (s? t:f=w1426:i32)
          }
          frame 16 {
            # "raise intake\nstop intaking"
            n682 = shared-variable ".\\Shared Variables.lvlib\\Driver.lvlib\\driverButton6"(FALSE ("driverButton1")) -> (error out=w1437:errorcluster)  [unwired: 1 in]
            n683 = shared-variable ".\\Shared Variables.lvlib\\Driver.lvlib\\driverButton1"(TRUE ("driverButton1"), error in=w1437) -> ()  [unwired: 1 out]
            n684 = Increment(x=w1440) -> (x+1=w1439:i32)
          }
          frame 17 {
            # "wait for intake to raise\nDelay for CMD"
            n685 = call "Delay.vi"("Timer Going?"=TRUE, "Time to Wait (ms)"=100.0) -> ("Time Up"=w1449:bool)
            n686 = Select(t=27, s=w1449, f=w1447) -> (s? t:f=w1446:i32)
          }
          frame 27 {
            # "wait for intake to raise\nDelay for CMD"
            n687 = shared-variable ".\\Shared Variables.lvlib\\Driver.lvlib\\driverButton1"(FALSE ("driverButton1")) -> (error out=w1452:errorcluster)  [unwired: 1 in]
            n688 = shared-variable ".\\Shared Variables.lvlib\\Misc..lvlib\\Desired Intake Speed"(0.2 ("Desired Intake Speed"), error in=w1452) -> ()  [unwired: 1 out]
            n689 = call "Delay.vi"("Timer Going?"=TRUE, "Time to Wait (ms)"=100.0) -> ("Time Up"=w1461:bool)
            n690 = Select(t=28, s=w1461, f=w1459) -> (s? t:f=w1458:i32)
          }
          frame 28 {
            # "Typically 250ms"
            # "wait for intake to raise\nDelay for CMD"
            n691 = shared-variable ".\\Shared Variables.lvlib\\Driver.lvlib\\driverButton6"(TRUE ("driverButton1")) -> ()  [unwired: 1 in, 1 out]
            n692 = call "Delay.vi"("Timer Going?"=TRUE, "Time to Wait (ms)"=500.0) -> ("Time Up"=w1471:bool)
            n693 = Select(t=20, s=w1471, f=w1469) -> (s? t:f=w1468:i32)
          }
          frame 20 {
            # "run intake motor\n lower intake"
            n694 = Increment(x=w1478) -> (x+1=w1477:i32)
            n695 = shared-variable ".\\Shared Variables.lvlib\\Driver.lvlib\\driverButton1"(TRUE ("driverButton1")) -> ()  [unwired: 1 in, 1 out]
          }
          frame 21 {
            # "Consider decreasing settling time"
            # "wait for intake to lower\n(450ms)"
            n696 = Increment(x=w1483) -> (x+1=w1486:i32)
            n697 = call "Delay.vi"("Timer Going?"=TRUE, "Time to Wait (ms)"=450.0 ("Wait for Intake to Lower (450ms)")) -> ("Time Up"=w1485:bool)
            n698 = Select(t=w1486, s=w1485, f=w1483) -> (s? t:f=w1482:i32)
          }
          frame 22 {
            # "stop running intake motor\nfire\nDe-Assert Lower Intake"
            n699 = Increment(x=w1492) -> (x+1=w1493:i32)
            n700 = Greater Or Equal?(x=w1488, y=w1491) -> (x >= y?=w1490:bool)
            n701 = Select(t=w1493, s=w1490, f=w1492) -> (s? t:f=w1494:i32)
            n702 = shared-variable ".\\Shared Variables.lvlib\\Driver.lvlib\\driverButton1"(FALSE ("driverButton1")) -> (error out=w1497:errorcluster)  [unwired: 1 in]
            n703 = shared-variable ".\\Shared Variables.lvlib\\Driver.lvlib\\driverButton6"(FALSE ("driverButton1"), error in=w1497) -> (error out=w1499:errorcluster)
            n704 = shared-variable ".\\Shared Variables.lvlib\\Driver.lvlib\\driverButton8"(TRUE ("driverButton1"), error in=w1499) -> ()  [unwired: 1 out]
          }
          frame 23 {
            # "wait for fire"
            n705 = Increment(x=w1507) -> (x+1=w1510:i32)
            n706 = call "Delay.vi"("Timer Going?"=TRUE, "Time to Wait (ms)"=w1502) -> ("Time Up"=w1509:bool)
            n707 = Select(t=w1510, s=w1509, f=w1507) -> (s? t:f=w1506:i32)
          }
          frame 24 {
            # "stop fire\nretract arm"
            n708 = shared-variable ".\\Shared Variables.lvlib\\Driver.lvlib\\driverButton8"(FALSE ("driverButton8")) -> (error out=w1514:errorcluster)  [unwired: 1 in]
            n709 = shared-variable ".\\Shared Variables.lvlib\\Driver.lvlib\\driverButton7"(TRUE ("driverButton8"), error in=w1514) -> ()  [unwired: 1 out]
            n710 = Increment(x=w1516) -> (x+1=w1515:i32)
          }
          frame 25 {
            # "wait for retract"
            n711 = call <vilib>:"WPI_AnalogChannelGetVoltage.vi"("AIDeviceRef"=w1522) -> ("Voltage"=w1526:dbl)  [unwired: 8 in, 2 out]
            n712 = In Range and Coerce(upper limit=5.0, x=w1526, lower limit=1.5) -> (In Range?=w1523:bool)  [unwired: 1 out]
            n713 = Increment(x=w1527) -> (x+1=w1529:i32)
            n714 = Select(t=w1529, s=w1523, f=w1527) -> (s? t:f=w1528:i32)
          }
          frame 26 {
            # "wait for fire"
            # "bring intake arm up\nEND AUTO"
            n715 = shared-variable ".\\Shared Variables.lvlib\\Driver.lvlib\\driverButton7"(FALSE ("driverButton8")) -> (error out=w1539:errorcluster)  [unwired: 1 in]
            n716 = shared-variable ".\\Shared Variables.lvlib\\Driver.lvlib\\driverButton1"(TRUE ("driverButton1"), error in=w1539) -> ()  [unwired: 1 out]
            n717 = call "Delay.vi"("Timer Going?"=TRUE, "Time to Wait (ms)"=50.0) -> ("Time Up"=w1533:bool)
            n718 = Select(t=29, s=w1533, f=w1531) -> (s? t:f=w1530:i32)
          }
          frame 29 {
            w1547 = 0.0 ("Desired Intake Speed")
            w1543 = FALSE ("driverButton1")
            n719 = shared-variable ".\\Shared Variables.lvlib\\Driver.lvlib\\driverButton1"(w1543) -> (error out=w1542:errorcluster)  [unwired: 1 in]
            n720 = shared-variable ".\\Shared Variables.lvlib\\Driver.lvlib\\driverButton6"(w1543, error in=w1542) -> ()  [unwired: 1 out]
            n721 = shared-variable ".\\Shared Variables.lvlib\\Misc..lvlib\\Desired Intake Speed"(w1547) -> (error out=w1546:errorcluster)  [unwired: 1 in]
            n722 = shared-variable ".\\Shared Variables.lvlib\\Driver.lvlib\\driverJoystickAxis3"(w1547, error in=w1546) -> (error out=w1545:errorcluster)
            n723 = shared-variable ".\\Shared Variables.lvlib\\Driver.lvlib\\driverJoystickAxis1"(w1547, error in=w1545) -> (error out=w1544:errorcluster)
            n724 = shared-variable ".\\Shared Variables.lvlib\\Driver.lvlib\\driverJoystickAxis2"(w1547, error in=w1544) -> ()  [unwired: 1 out]
          }
        }
        n725 = Select(t=cluster{"output high":dbl, "output low":dbl} {"output high"=0.0, "output low"=0.0} ("output range"), s=w1188, f=cluster{"output high":dbl, "output low":dbl} {"output high"=0.6, "output low"=-0.6} ("output range")) -> (s? t:f=w1189:cluster{"output high":dbl, "output low":dbl})
        n726 = call-poly <vilib>:"PID.vi"("reinitialize? (F)"=w1188, "output range"=w1189, "PID gains"=w1195, "process variable"=w1187, "setpoint"=w1196) -> ("output"=w1198:dbl)  [unwired: 5 in, 1 out]
        n727 = shared-variable ".\\Shared Variables.lvlib\\Driver.lvlib\\driverJoystickAxis3"(w1198) -> ()  [unwired: 1 in, 1 out]
        "State 5" <- w1197
      }
    }
    frame 4 {
      n728 = Divide(x=250.0, y=360.0) -> (x/y=w1556:dbl)
      n729 = Multiply(x="auto 3 distance 4", y=w1556) -> (x*y=w1558:dbl)
      n730 = call <vilib>:"WPI_EncoderRefNum Registry Get.vi"("refnum name"="leftWheelEncoder") -> ("EncoderDevRef"=w1575:T3)  [unwired: 9 in, 1 out]
      n731 = call <vilib>:"WPI_EncoderRefNum Registry Get.vi"("refnum name"="rightWheelEncoder") -> ("EncoderDevRef"=w1574:T3)  [unwired: 9 in, 1 out]
      n732 = call <vilib>:"WPI_GyroRefNum Registry Get.vi"("refnum name"="yawGyro") -> ("error out"=w1562:errorcluster, "GyroDevRef"=w1563:T7)  [unwired: 9 in]
      n733 = Select(t=w1558, s=w1553, f="auto 3 distance 4") -> (s? t:f=w1552:dbl)
      n734 = call <vilib>:"WPI_GyroReset.vi"("error in (no error)"=w1562, "GyroDevRef"=w1563) -> ("GyroDevRef"=w1560:T7)  [unwired: 8 in, 1 out]
      n735 = call <vilib>:"WPI_EncoderReset.vi"("EncoderDevRef"=w1575) -> ("EncoderDevRef"=w1571:T3)  [unwired: 9 in, 1 out]
      n736 = call <vilib>:"WPI_AnalogChannelRefNum Registry Get.vi"("refnum name"="irProximDistCatapult") -> ("AIDeviceRef"=w1569:T10)  [unwired: 9 in, 1 out]
      n737 = call <vilib>:"WPI_AnalogChannelRefNum Registry Get.vi"("refnum name"="irProximDistCatDown") -> ("AIDeviceRef"=w1565:T10)  [unwired: 9 in, 1 out]
      n738 = call <vilib>:"WPI_EncoderReset.vi"("EncoderDevRef"=w1574) -> ("EncoderDevRef"=w1570:T3)  [unwired: 9 in, 1 out]
      n739 = while {
        tunnel: w1571 -> [w1592]
        tunnel: w1570 -> [w1591]
        tunnel: w1569 -> [w1586]
        shift-right: [w1585] -> _
        shift-left: 0 -> [w1584]
        tunnel: w1565 -> [w1583]
        tunnel: w1564 -> [w1581]
        tunnel: w1560 -> [_]
        tunnel: w1559 -> [w1578]
        tunnel: w1552 -> [w1577]
        stop <- FALSE stop-if-true
        n740 = shared-variable ".\\Shared Variables.lvlib\\Sensors-Actuators.lvlib\\Gyro.lvlib\\yawGyro"() -> (w1580:dbl)  [unwired: 1 in, 1 out]
        n741 = Wait (ms)(milliseconds to wait=u32 25) -> ()  [unwired: 1 out]
        n742 = case shown="7" w1584 {
          selector: w1584 -> [w1596 w1601 w1612 w1621 w1628 w1639 w1646 w1656 w1694 _ w1717 w1725 w1730 w1736 w1744 w1756 w1766 w1772 w1785 w1790 w1800 w1805 w1813 w1820 w1830 w1837 w1846 w1856 w1864 w1868 w1879 w1889 w1894 w1903 w1911]
          tunnel: [w1595 w1604 w1613 w1619 w1631 w1638 w1645 w1665 w1701 3 w1716 w1726 w1729 w1735 w1743 w1755 w1765 w1770 w1784 w1789 w1799 w1804 w1812 w1819 w1829 w1836 w1845 w1857 w1863 w1869 w1878 w1887 w1893 w1902 w1911] -> w1585
          tunnel: w1592 -> [_ _ _ _ _ _ _ w1667 w1703 _ w1715 _ _ _ _ _ _ _ _ _ _ _ _ _ _ _ _ _ _ _ _ _ _ _ _]
          tunnel: w1591 -> [_ _ _ _ _ _ _ w1666 w1702 _ w1714 _ _ _ _ _ _ _ _ _ _ _ _ _ _ _ _ _ _ _ _ _ _ _ _]
          tunnel: w1586 -> [_ _ _ _ _ _ _ _ _ _ _ _ _ _ _ _ _ w1779 _ _ _ _ _ _ _ _ _ _ _ _ _ _ _ _ _]
          tunnel: w1583 -> [_ _ _ _ _ _ _ _ _ _ _ _ _ _ _ w1754 _ _ _ _ _ _ _ _ _ _ _ w1851 _ _ _ _ _ _ _]
          tunnel: [0.0 ("setpoint") 0.0 ("setpoint") 0.0 ("setpoint") 0.0 ("setpoint") 0.0 ("setpoint") 0.0 ("setpoint") 0.0 ("setpoint") 0.0 ("setpoint") 0.0 ("setpoint") 0.0 ("setpoint") 0.0 ("setpoint") 0.0 ("setpoint") w1728 w1734 w1742 w1749 w1762 w1769 w1781 w1788 w1796 w1803 w1811 w1818 w1826 w1835 w1843 w1850 w1860 w1867 w1875 0.0 ("Double") w1892 w1907 w1910] -> w1582
          tunnel: w1581 -> [_ _ _ _ _ _ _ _ _ _ _ _ _ _ _ _ _ _ _ _ _ _ _ _ _ _ _ _ _ _ _ _ _ _ _]
          tunnel: w1580 -> [_ _ _ _ _ _ _ _ _ _ _ _ w1728 w1734 w1742 w1749 w1762 w1769 w1781 w1788 w1796 w1803 w1811 w1818 w1826 w1835 w1843 w1850 w1860 w1867 w1875 _ w1892 w1907 w1910]
          tunnel: [FALSE FALSE FALSE FALSE FALSE FALSE FALSE FALSE FALSE FALSE FALSE TRUE TRUE FALSE FALSE FALSE FALSE FALSE FALSE FALSE FALSE FALSE FALSE FALSE FALSE FALSE FALSE FALSE FALSE FALSE FALSE FALSE FALSE FALSE FALSE] -> w1579
          tunnel: w1577 -> [_ _ _ _ _ _ _ w1651 w1689 _ _ _ _ _ _ _ _ _ _ _ _ _ _ _ _ _ _ _ _ _ _ _ _ _ _]
          frame 0, Default {
            # "switch to manual"
            n743 = shared-variable ".\\Shared Variables.lvlib\\Driver.lvlib\\driverButton10"(TRUE ("driverButton10")) -> ()  [unwired: 1 in, 1 out]
            n744 = Increment(x=w1596) -> (x+1=w1595:i32)
          }
          frame 1 {
            # "delay\nset intake speed"
            n745 = shared-variable ".\\Shared Variables.lvlib\\Misc..lvlib\\Desired Intake Speed"(0.2 ("Intake RPM")) -> ()  [unwired: 1 in, 1 out]
            n746 = Increment(x=w1601) -> (x+1=w1602:i32)
            n747 = call "Delay.vi"("Timer Going?"=TRUE, "Time to Wait (ms)"=100.0) -> ("Time Up"=w1605:bool)
            n748 = Select(t=w1602, s=w1605, f=w1601) -> (s? t:f=w1604:i32)
          }
          frame 2 {
            # "turn manual variable false\nrun intake\nopen intake"
            n749 = disable-structure shown="Disabled" {
              disable-tunnel: [w1615 _] -> _
              frame Disabled {
                n750 = shared-variable ".\\Shared Variables.lvlib\\Driver.lvlib\\driverButton10"(FALSE ("driverButton10")) -> (error out=w1615:errorcluster)  [unwired: 1 in]
              }
              frame Enabled {
              }
            }
            n751 = shared-variable ".\\Shared Variables.lvlib\\Driver.lvlib\\driverButton6"(TRUE ("driverButton6")) -> (error out=w1610:errorcluster)  [unwired: 1 in]
            n752 = shared-variable ".\\Shared Variables.lvlib\\Driver.lvlib\\driverButton1"(TRUE ("driverButton1"), error in=w1610) -> ()  [unwired: 1 out]
            n753 = Add(x=2, y=w1612) -> (x+y=w1613:i32)
          }
          frame 3 {
            n754 = call "Delay.vi"("Timer Going?"=TRUE, "Time to Wait (ms)"=150.0) -> ("Time Up"=w1624:bool)
            n755 = Add(x=26, y=w1621) -> (x+y=w1622:i32)
            n756 = Select(t=w1622, s=w1624, f=w1621) -> (s? t:f=w1619:i32)
          }
          frame 4 {
            # "wait for intake"
            n757 = Increment(x=w1628) -> (x+1=w1629:i32)
            n758 = call "Delay.vi"("Timer Going?"=TRUE, "Time to Wait (ms)"=500.0) -> ("Time Up"=w1632:bool)
            n759 = Select(t=w1629, s=w1632, f=w1628) -> (s? t:f=w1631:i32)
          }
          frame 5 {
            # "turn intake off\nset intake speed"
            n760 = shared-variable ".\\Shared Variables.lvlib\\Driver.lvlib\\driverButton6"(FALSE ("driverButton6")) -> (error out=w1640:errorcluster)  [unwired: 1 in]
            n761 = shared-variable ".\\Shared Variables.lvlib\\Misc..lvlib\\Desired Intake Speed"(1.0 ("Desired Intake Speed"), error in=w1640) -> (error out=w1636:errorcluster)
            n762 = shared-variable ".\\Shared Variables.lvlib\\Driver.lvlib\\driverButton1"(FALSE ("driverButton1"), error in=w1636) -> ()  [unwired: 1 out]
            n763 = Increment(x=w1639) -> (x+1=w1638:i32)
          }
          frame 6 {
            # "wait for variables"
            n764 = Increment(x=w1646) -> (x+1=w1647:i32)
            n765 = call "Delay.vi"("Timer Going?"=TRUE, "Time to Wait (ms)"=100.0) -> ("Time Up"=w1649:bool)
            n766 = Select(t=w1647, s=w1649, f=w1646) -> (s? t:f=w1645:i32)
          }
          frame 7 {
            # "run intake\ndrive"
            n767 = call <vilib>:"WPI_EncoderGet.vi"("EncoderDevRef"=w1667) -> ("Distance"=w1664:dbl)  [unwired: 5 in, 5 out]
            n768 = call <vilib>:"WPI_EncoderGet.vi"("EncoderDevRef"=w1666) -> ("Distance"=w1663:dbl)  [unwired: 5 in, 5 out]
            n769 = Add(x=w1664, y=w1663) -> (x+y=w1662:dbl)
            n770 = shared-variable ".\\Shared Variables.lvlib\\Driver.lvlib\\driverButton6"(TRUE ("driverButton6")) -> (error out=w1654:errorcluster)  [unwired: 1 in]
            n771 = Divide(x=w1662, y=2.0) -> (x/y=w1660:dbl)
            n772 = Greater?(x=w1660, y=w1651) -> (0:w1659:bool)
            n773 = Increment(x=w1656) -> (x+1=w1657:i32)
            n774 = Select(t=w1657, s=w1659, f=w1656) -> (s? t:f=w1665:i32)
            n775 = shared-variable ".\\Shared Variables.lvlib\\Driver.lvlib\\driverJoystickAxis2"(-0.8 ("driverJoystickAxis2"), error in=w1654) -> ()  [unwired: 1 out]
          }
          frame 33 {
            # "Must put in not to exceed\nvalue for Encoder!!"
            # "run intake\ndrive Back for Ball 3\nTrack X"
            n776 = call <vilib>:"WPI_EncoderGet.vi"("EncoderDevRef"=w1703) -> ("Distance"=w1700:dbl)  [unwired: 5 in, 5 out]
            n777 = call <vilib>:"WPI_EncoderGet.vi"("EncoderDevRef"=w1702) -> ("Distance"=w1699:dbl)  [unwired: 5 in, 5 out]
            n778 = Add(x=w1700, y=w1699) -> (x+y=w1698:dbl)
            n779 = shared-variable ".\\Shared Variables.lvlib\\Vision.lvlib\\Ball X Time"() -> (w1668:dbl)  [unwired: 1 in, 1 out]
            n780 = shared-variable ".\\Shared Variables.lvlib\\Sensors-Actuators.lvlib\\in intake"() -> (w1688:bool)  [unwired: 1 in, 1 out]
            n781 = shared-variable ".\\Shared Variables.lvlib\\Vision.lvlib\\Ball X"() -> (w1671:dbl)  [unwired: 1 in, 1 out]
            n782 = shared-variable ".\\Shared Variables.lvlib\\Vision.lvlib\\Valid Ball"() -> (w1678:bool)  [unwired: 1 in, 1 out]
            n783 = Increment(x=w1694) -> (x+1=w1695:i32)
            n784 = Divide(x=w1698, y=2.0) -> (x/y=w1696:dbl)
            n785 = Greater?(x=w1696, y=w1689) -> ()  [unwired: 1 out]
            n786 = Select(t=w1695, s=w1688, f=w1694) -> (s? t:f=w1701:i32)
            n787 = call "Rate Selective Filter.vi"("Hyster"=0.3, "Rate Thresh"="Rate Thresh", "hi limit"=50.0, "lo limit"=-100.0, "Time"=w1668, "Distance"=w1671) -> ("Filtered"=w1670:dbl)  [unwired: 1 in, 2 out]
            n788 = shared-variable ".\\Shared Variables.lvlib\\Driver.lvlib\\driverButton6"(TRUE ("driverButton6")) -> (error out=w1692:errorcluster)  [unwired: 1 in]
            n789 = Select(t=0.5 ("driverJoystickAxis2"), s=w1678, f=0.0) -> (s? t:f=w1675:dbl)
            n790 = shared-variable ".\\Shared Variables.lvlib\\Driver.lvlib\\driverJoystickAxis2"(w1675, error in=w1692) -> ()  [unwired: 1 out]
            n791 = In Range and Coerce(upper limit=7.0, x=w1670, lower limit=-7.0) -> (In Range?=w1679:bool)  [unwired: 1 out]
            n792 = call-poly <vilib>:"PID.vi"("output range"=cluster{"output high":dbl, "output low":dbl} {"output high"=1.0, "output low"=-1.0}, "PID gains"="Track PID", "process variable"=w1670, "setpoint"=0.0) -> ("output"=w1686:dbl)  [unwired: 6 in, 1 out]
            n793 = Select(t=0.0, s=w1679, f=w1686) -> (s? t:f=w1680:dbl)
            n794 = shared-variable ".\\Shared Variables.lvlib\\Driver.lvlib\\driverJoystickAxis1"(w1680) -> ()  [unwired: 1 in, 1 out]
          }
          frame 8 {
            # "stop drive"
            n795 = shared-variable ".\\Shared Variables.lvlib\\Driver.lvlib\\driverJoystickAxis2"(0.0 ("driverJoystickAxis2")) -> ()  [unwired: 1 in, 1 out]
          }
          frame 9 {
            # "wait for encoder to stop"
            n796 = call <vilib>:"WPI_EncoderGet.vi"("EncoderDevRef"=w1715) -> ("Stopped"=w1713:bool)  [unwired: 5 in, 5 out]
            n797 = call <vilib>:"WPI_EncoderGet.vi"("EncoderDevRef"=w1714) -> ("Stopped"=w1712:bool)  [unwired: 5 in, 5 out]
            n798 = And(x=w1713, y=w1712) -> (x .and. y?=w1711:bool)
            n799 = Select(t=32, s=w1711, f=w1717) -> (s? t:f=w1716:i32)
          }
          frame 32 {
            n800 = shared-variable ".\\Shared Variables.lvlib\\Driver.lvlib\\driverJoystickAxis1"(0.0 ("setpoint")) -> ()  [unwired: 1 in, 1 out]
            n801 = call "Delay.vi"("Timer Going?"=TRUE, "Time to Wait (ms)"=2000.0) -> ("Time Up"=w1720:bool)
            n802 = Select(t=10, s=w1720, f=w1725) -> (s? t:f=w1726:i32)
          }
          frame 10 {
            # "fire"
            n803 = disable-structure shown="Disabled" {
              frame Disabled {
                n804 = shared-variable ".\\Shared Variables.lvlib\\Driver.lvlib\\driverJoystickAxis1"(0.0 ("driverJoystickAxis1")) -> ()  [unwired: 1 in, 1 out]
              }
              frame Enabled {
              }
            }
            n805 = shared-variable ".\\Shared Variables.lvlib\\Driver.lvlib\\driverButton8"(TRUE ("driverButton8")) -> ()  [unwired: 1 in, 1 out]
            n806 = Increment(x=w1730) -> (x+1=w1729:i32)
          }
          frame 11 {
            # "wait for fire to comlete"
            n807 = Increment(x=w1736) -> (x+1=w1738:i32)
            n808 = call "Delay.vi"("Timer Going?"=TRUE, "Time to Wait (ms)"=500.0) -> ("Time Up"=w1739:bool)
            n809 = Select(t=w1738, s=w1739, f=w1736) -> (s? t:f=w1735:i32)
          }
          frame 12 {
            # "stop fire\nretract arm"
            n810 = shared-variable ".\\Shared Variables.lvlib\\Driver.lvlib\\driverButton8"(FALSE ("driverButton8")) -> (error out=w1745:errorcluster)  [unwired: 1 in]
            n811 = shared-variable ".\\Shared Variables.lvlib\\Driver.lvlib\\driverButton7"(TRUE ("driverButton8"), error in=w1745) -> ()  [unwired: 1 out]
            n812 = Increment(x=w1744) -> (x+1=w1743:i32)
          }
          frame 13 {
            # "wait for arm to come down"
            n813 = disable-structure shown="Disabled" {
              disable-tunnel: [w1759 _] -> _
              frame Disabled {
                n814 = call "Delay.vi"("Timer Going?"=TRUE, "Time to Wait (ms)"=1000.0) -> ("Time Up"=w1759:bool)
              }
              frame Enabled {
              }
            }
            n815 = call <vilib>:"WPI_AnalogChannelGetVoltage.vi"("AIDeviceRef"=w1754) -> ("Voltage"=w1753:dbl)  [unwired: 8 in, 2 out]
            n816 = Increment(x=w1756) -> (x+1=w1757:i32)
            n817 = In Range and Coerce(upper limit=5.0, x=w1753, lower limit=1.5) -> (In Range?=w1750:bool)  [unwired: 1 out]
            n818 = Select(t=w1757, s=w1750, f=w1756) -> (s? t:f=w1755:i32)
          }
          frame 14 {
            # "intake ball 2"
            n819 = Increment(x=w1766) -> (x+1=w1765:i32)
            n820 = shared-variable ".\\Shared Variables.lvlib\\Driver.lvlib\\driverButton7"(FALSE ("driverButton8")) -> (error out=w1763:errorcluster)  [unwired: 1 in]
            n821 = shared-variable ".\\Shared Variables.lvlib\\Driver.lvlib\\driverButton6"(TRUE ("driverButton1"), error in=w1763) -> ()  [unwired: 1 out]
          }
          frame 15 {
            # "wait for intake to finish"
            n822 = call <vilib>:"WPI_AnalogChannelGetVoltage.vi"("AIDeviceRef"=w1779) -> ("Voltage"=w1778:dbl)  [unwired: 8 in, 2 out]
            n823 = In Range and Coerce(upper limit=5.0, x=w1778, lower limit=0.56) -> (In Range?=w1775:bool)  [unwired: 1 out]
            n824 = call "Stable.vi"("Eval Period (sec)"=0.2, "Signal Input"=w1775) -> ("Stable"=w1773:bool)  [unwired: 9 in]
            n825 = Increment(x=w1772) -> (x+1=w1771:i32)
            n826 = Select(t=w1771, s=w1773, f=w1772) -> (s? t:f=w1770:i32)
          }
          frame 16 {
            # "raise intake\nstop intakign"
            n827 = shared-variable ".\\Shared Variables.lvlib\\Driver.lvlib\\driverButton6"(FALSE ("driverButton1")) -> (error out=w1782:errorcluster)  [unwired: 1 in]
            n828 = shared-variable ".\\Shared Variables.lvlib\\Driver.lvlib\\driverButton1"(TRUE ("driverButton1"), error in=w1782) -> ()  [unwired: 1 out]
            n829 = Increment(x=w1785) -> (x+1=w1784:i32)
          }
          frame 17 {
            # "wait for intake to raise"
            n830 = Increment(x=w1790) -> (x+1=w1793:i32)
            n831 = call "Delay.vi"("Timer Going?"=TRUE, "Time to Wait (ms)"=400.0) -> ("Time Up"=w1792:bool)
            n832 = Select(t=w1793, s=w1792, f=w1790) -> (s? t:f=w1789:i32)
          }
          frame 18 {
            # "make variable false"
            n833 = Increment(x=w1800) -> (x+1=w1799:i32)
            n834 = shared-variable ".\\Shared Variables.lvlib\\Driver.lvlib\\driverButton1"(FALSE ("driverButton1")) -> (error out=w1797:errorcluster)  [unwired: 1 in]
            n835 = shared-variable ".\\Shared Variables.lvlib\\Misc..lvlib\\Desired Intake Speed"(0.2 ("Desired Intake Speed"), error in=w1797) -> ()  [unwired: 1 out]
          }
          frame 19 {
            # "variable delay"
            n836 = Increment(x=w1805) -> (x+1=w1808:i32)
            n837 = call "Delay.vi"("Timer Going?"=TRUE, "Time to Wait (ms)"=50.0) -> ("Time Up"=w1807:bool)
            n838 = Select(t=w1808, s=w1807, f=w1805) -> (s? t:f=w1804:i32)
          }
          frame 20 {
            # "run intake motor lower intake"
            n839 = Increment(x=w1813) -> (x+1=w1812:i32)
            n840 = shared-variable ".\\Shared Variables.lvlib\\Driver.lvlib\\driverButton6"(TRUE ("driverButton1")) -> (error out=w1814:errorcluster)  [unwired: 1 in]
            n841 = shared-variable ".\\Shared Variables.lvlib\\Driver.lvlib\\driverButton1"(TRUE ("driverButton1"), error in=w1814) -> ()  [unwired: 1 out]
          }
          frame 21 {
            # "wait for intake to lower"
            n842 = Increment(x=w1820) -> (x+1=w1823:i32)
            n843 = call "Delay.vi"("Timer Going?"=TRUE, "Time to Wait (ms)"=400.0) -> ("Time Up"=w1822:bool)
            n844 = Select(t=w1823, s=w1822, f=w1820) -> (s? t:f=w1819:i32)
          }
          frame 22 {
            # "stop runnint intake motor\nfire"
            n845 = Increment(x=w1830) -> (x+1=w1829:i32)
            n846 = shared-variable ".\\Shared Variables.lvlib\\Driver.lvlib\\driverButton1"(FALSE ("driverButton1")) -> (error out=w1827:errorcluster)  [unwired: 1 in]
            n847 = shared-variable ".\\Shared Variables.lvlib\\Driver.lvlib\\driverButton6"(FALSE ("driverButton1"), error in=w1827) -> (error out=w1831:errorcluster)
            n848 = shared-variable ".\\Shared Variables.lvlib\\Driver.lvlib\\driverButton8"(TRUE ("driverButton1"), error in=w1831) -> ()  [unwired: 1 out]
          }
          frame 23 {
            # "wait for fire"
            n849 = Increment(x=w1837) -> (x+1=w1840:i32)
            n850 = call "Delay.vi"("Timer Going?"=TRUE, "Time to Wait (ms)"=400.0) -> ("Time Up"=w1839:bool)
            n851 = Select(t=w1840, s=w1839, f=w1837) -> (s? t:f=w1836:i32)
          }
          frame 24 {
            # "Release Fire"
            # "Retract Shooter"
            # "stop fire\nretract arm"
            n852 = shared-variable ".\\Shared Variables.lvlib\\Driver.lvlib\\driverButton8"(FALSE ("driverButton8")) -> (error out=w1844:errorcluster)  [unwired: 1 in]
            n853 = shared-variable ".\\Shared Variables.lvlib\\Driver.lvlib\\driverButton7"(TRUE ("driverButton8"), error in=w1844) -> ()  [unwired: 1 out]
            n854 = Increment(x=w1846) -> (x+1=w1845:i32)
          }
          frame 25 {
            # "wait for retract"
            n855 = Increment(x=w1856) -> (x+1=w1858:i32)
            n856 = call <vilib>:"WPI_AnalogChannelGetVoltage.vi"("AIDeviceRef"=w1851) -> ("Voltage"=w1855:dbl)  [unwired: 8 in, 2 out]
            n857 = In Range and Coerce(upper limit=5.0, x=w1855, lower limit=1.5) -> (In Range?=w1852:bool)  [unwired: 1 out]
            n858 = Select(t=w1858, s=w1852, f=w1856) -> (s? t:f=w1857:i32)
          }
          frame 26 {
            # "**"
            # "Intake Up"
            # "Release Retract"
            # "bring intake arm up"
            n859 = shared-variable ".\\Shared Variables.lvlib\\Driver.lvlib\\driverButton7"(FALSE ("driverButton8")) -> (error out=w1861:errorcluster)  [unwired: 1 in]
            n860 = shared-variable ".\\Shared Variables.lvlib\\Driver.lvlib\\driverButton1"(FALSE ("driverButton1"), error in=w1861) -> ()  [unwired: 1 out]
            n861 = Increment(x=w1864) -> (x+1=w1863:i32)
          }
          frame 27 {
            # "wait for intake to rise"
            n862 = Increment(x=w1868) -> (x+1=w1872:i32)
            n863 = call "Delay.vi"("Timer Going?"=TRUE, "Time to Wait (ms)"=400.0) -> ("Time Up"=w1871:bool)
            n864 = Select(t=w1872, s=w1871, f=w1868) -> (s? t:f=w1869:i32)
          }
          frame 28 {
            # "Stop Intake Motor"
            # "Release Intake"
            # "set intake false"
            n865 = shared-variable ".\\Shared Variables.lvlib\\Driver.lvlib\\driverButton1"(FALSE ("driverButton1")) -> (error out=w1880:errorcluster)  [unwired: 1 in]
            n866 = shared-variable ".\\Shared Variables.lvlib\\Misc..lvlib\\Desired Intake Speed"(0.0 ("Desired Intake Speed"), error in=w1880) -> (error out=w1877:errorcluster)
            n867 = disable-structure shown="Disabled" {
              disable-tunnel: w1877 -> [w1883 _]
              frame Disabled {
                n868 = shared-variable ".\\Shared Variables.lvlib\\Driver.lvlib\\driverButton10"(TRUE ("driverButton10"), error in=w1883) -> ()  [unwired: 1 out]
              }
              frame Enabled {
              }
            }
            n869 = Add(x=2, y=w1879) -> (x+y=w1878:i32)
          }
          frame 29 {
            # "stop intake roller"
            n870 = shared-variable ".\\Shared Variables.lvlib\\Driver.lvlib\\driverButton6"(FALSE ("driverButton6")) -> ()  [unwired: 1 in, 1 out]
            n871 = Subtract(x=w1889, y=20) -> (x-y=w1887:i32)
          }
          frame 30 {
            n872 = Increment(x=w1894) -> (x+1=w1895:i32)
            n873 = call "Delay.vi"("Timer Going?"=TRUE, "Time to Wait (ms)"=250.0) -> ("Time Up"=w1897:bool)
            n874 = Select(t=w1895, s=w1897, f=w1894) -> (s? t:f=w1893:i32)
          }
          frame 31 {
            n875 = call "Delay.vi"("Timer Going?"=TRUE, "Time to Wait (ms)"=20.0) -> ("Time Up"=w1899:bool)
            n876 = Add(x=w1903, y=2) -> (x+y=w1904:i32)
            n877 = Select(t=w1904, s=w1899, f=w1903) -> (s? t:f=w1902:i32)
          }
          frame 34 {
            w1908 = 0.0 ("driverJoystickAxis2")
            n878 = shared-variable ".\\Shared Variables.lvlib\\Driver.lvlib\\driverJoystickAxis2"(w1908) -> ()  [unwired: 1 in, 1 out]
            n879 = shared-variable ".\\Shared Variables.lvlib\\Driver.lvlib\\driverJoystickAxis1"(w1908) -> ()  [unwired: 1 in, 1 out]
          }
        }
        n880 = call-poly <vilib>:"PID.vi"("reinitialize? (F)"=w1579, "output range"=cluster{"output high":dbl, "output low":dbl} {"output high"=0.75, "output low"=-0.75}, "PID gains"=w1578, "process variable"=w1580, "setpoint"=w1582) -> ("output"=w1587:dbl)  [unwired: 5 in, 1 out]
        n881 = shared-variable ".\\Shared Variables.lvlib\\Driver.lvlib\\driverJoystickAxis3"(w1587) -> ()  [unwired: 1 in, 1 out]
        "State" <- w1584
      }
    }
    frame 8 {
      n882 = while {
        stop <- FALSE stop-if-true
        w1923 = T14 11 items=["HipCenter", "Spine", "ShoulderCenter", "Head", "ShoulderLeft", "ElbowLeft", "WristLeft", "HandLeft", "ShoulderRight", "ElbowRight", "WristRight", "HandRight", "HipLeft", "KneeLeft", "AnkleLeft", "FootLeft", "HipRight", "KneeRight", "AnkleRight", "FootRight"] ("Skeleton Joints")
        w1924 = T14 7 items=["HipCenter", "Spine", "ShoulderCenter", "Head", "ShoulderLeft", "ElbowLeft", "WristLeft", "HandLeft", "ShoulderRight", "ElbowRight", "WristRight", "HandRight", "HipLeft", "KneeLeft", "AnkleLeft", "FootLeft", "HipRight", "KneeRight", "AnkleRight", "FootRight"] ("Skeleton Joints")
        n883 = Wait (ms)(milliseconds to wait=u32 50) -> ()  [unwired: 1 out]
        n884 = call <vilib>:"WPI_DriverStationGet Kinect Vertices.vi"() -> ("Skeleton Vertices"=w1925:cluster{"x":sgl, "y":sgl, "z":sgl}[])  [unwired: 10 in, 1 out]
        n885 = Index Array(array=w1925, index #1=w1924, index #2=w1923) -> (element #1=w1922:cluster{"x":sgl, "y":sgl, "z":sgl}, element #2=w1921:cluster{"x":sgl, "y":sgl, "z":sgl})
        n886 = Subtract(x=w1922, y=w1921) -> (x-y=w1919:cluster{"x":sgl, "y":sgl, "z":sgl})
        n887 = Absolute Value(x=w1919) -> (abs(x)=→"x-y 2":cluster{"x":sgl, "y":sgl, "z":sgl})
        n888 = Unbundle(w1919) -> ("x"=w1913:sgl)  [unwired: 2 out]
        n889 = Absolute Value(x=w1913) -> (abs(x)=w1918:sgl)
        "Y" <- w1918
        n890 = Greater?(x=w1918, y="Threshhold 2") -> (0:w1916:bool)
        "x > y?" <- w1916
        n891 = shared-variable ".\\Shared Variables.lvlib\\Dashboard Variables.lvlib\\Kinect Status"(w1916) -> ()  [unwired: 1 in, 1 out]
      }
    }
  }
  "Autonomous state" <- w13
